vi "Server.vi"() -> ()   [LabVIEW 2020]
panel:
  in  "Door Stop":bool
  out "Open Door":bool
  out "Fire Alarm":bool
  out "AC4":bool
  out "AC3":bool
  out "AC2":bool
  out "AC1":bool
  out "KCW1":dbl(slide) scale=0.0..100.0
  out "KCW2":dbl(slide) scale=0.0..100.0
  out "B3W2":dbl(slide) scale=0.0..100.0
  out "B3W1":dbl(slide) scale=0.0..100.0
  out "B2W2":dbl(slide) scale=0.0..100.0
  out "B2W1":dbl(slide) scale=0.0..100.0
  out "LAW":dbl(slide) scale=0.0..100.0
  out "MBW":dbl(slide) scale=0.0..100.0
  out "MBC":bool
  out "B1C":bool
  out "MDC":bool
  out "B2C":bool
  out "B3C":bool
  out "TBC":bool
  out "SLC":bool
  out "B3O":bool
  out "B1O":bool
  out "LA":bool
  out "MBO":bool
  out "B2O":bool
  out "MDO":bool
  out "SLO":bool
  out "TBO":bool
  out "B3L2":bool
  out "B3L1":bool
  out "LL":bool
  out "B2WICL":bool
  out "B2L2":bool
  out "B2L1":bool
  out "MBL2":bool
  out "MBL1":bool
  out "GL2":bool
  out "GL1":bool
  out "MBWICL":bool
  out "MBL":bool
  out "KL2":bool
  out "KL1":bool
  out "TBL":bool
  out "SLL1":bool
  out "SLL2":bool
  out "DAL2":bool
  out "DAL1":bool
  out "LAL2":bool
  out "LAL1":bool
  out "PL":bool
  out "Brightness\nMaster Bath \nLight":u8
  out "Brightness\nKitchen \nLight 1":u8
  out "Brightness\nKitchen \nLight 2":u8
  out "Brightness\nService Laundry \nLight 1":u8
  out "Brightness\nService Laundry \nLight 2":u8
  out "Brightness\nT&B Light":u8
  out "Brightness\nMaster Bedroom \nLight 2":u8
  out "Brightness\nMaster Bedroom \nW.I.C. Light":u8
  out "Brightness\nLiving Area Light 1":u8
  out "Brightness\nLiving Area Light 2":u8
  out "Brightness\n Porch Light":u8
  out "Brightness\nBedroom 2 \nLight 2":u8
  out "Brightness\nBedroom 2 \nLight 1":u8
  out "Brightness\nLanai Light":u8
  out "Brightness\nDining Area Light 2":u8
  out "Brightness\nDining Area Light 1":u8
  out "Brightness\nGarage Light 2":u8
  out "Brightness\nGarage Light 1":u8
  out "Brightness\nBedroom 3 \nLight 2":u8
  out "Brightness\nBedroom 3 \nLight 1":u8
  out "Brightness\nBedroom 2 \nW.I.C. Light":u8
  out "Temperature":u8
  out "Brightness\nMaster Bedroom \nLight 1":u8
  in  "Alarm Stop":bool
  in  "Holiday Stop":bool
  in  "TV Living Area":refnum<k7>(container)
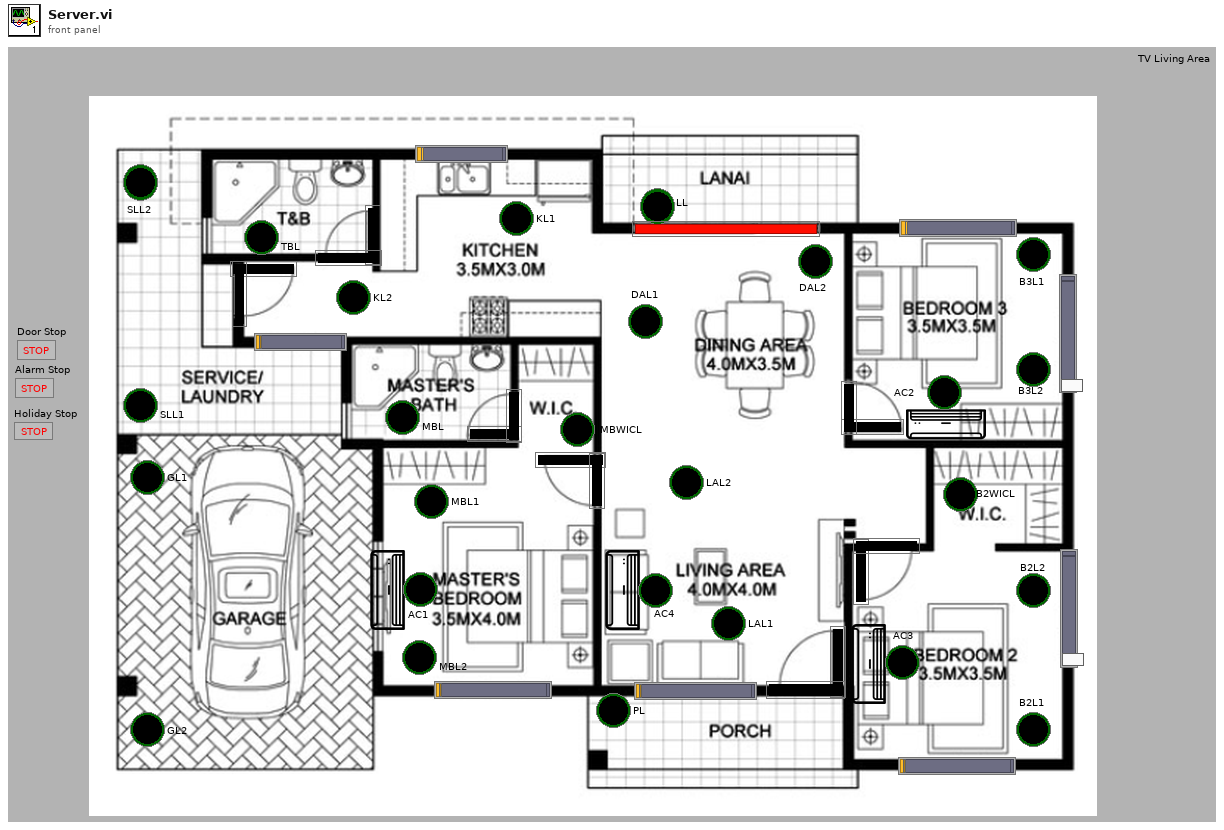
[diagram p1: front panel]
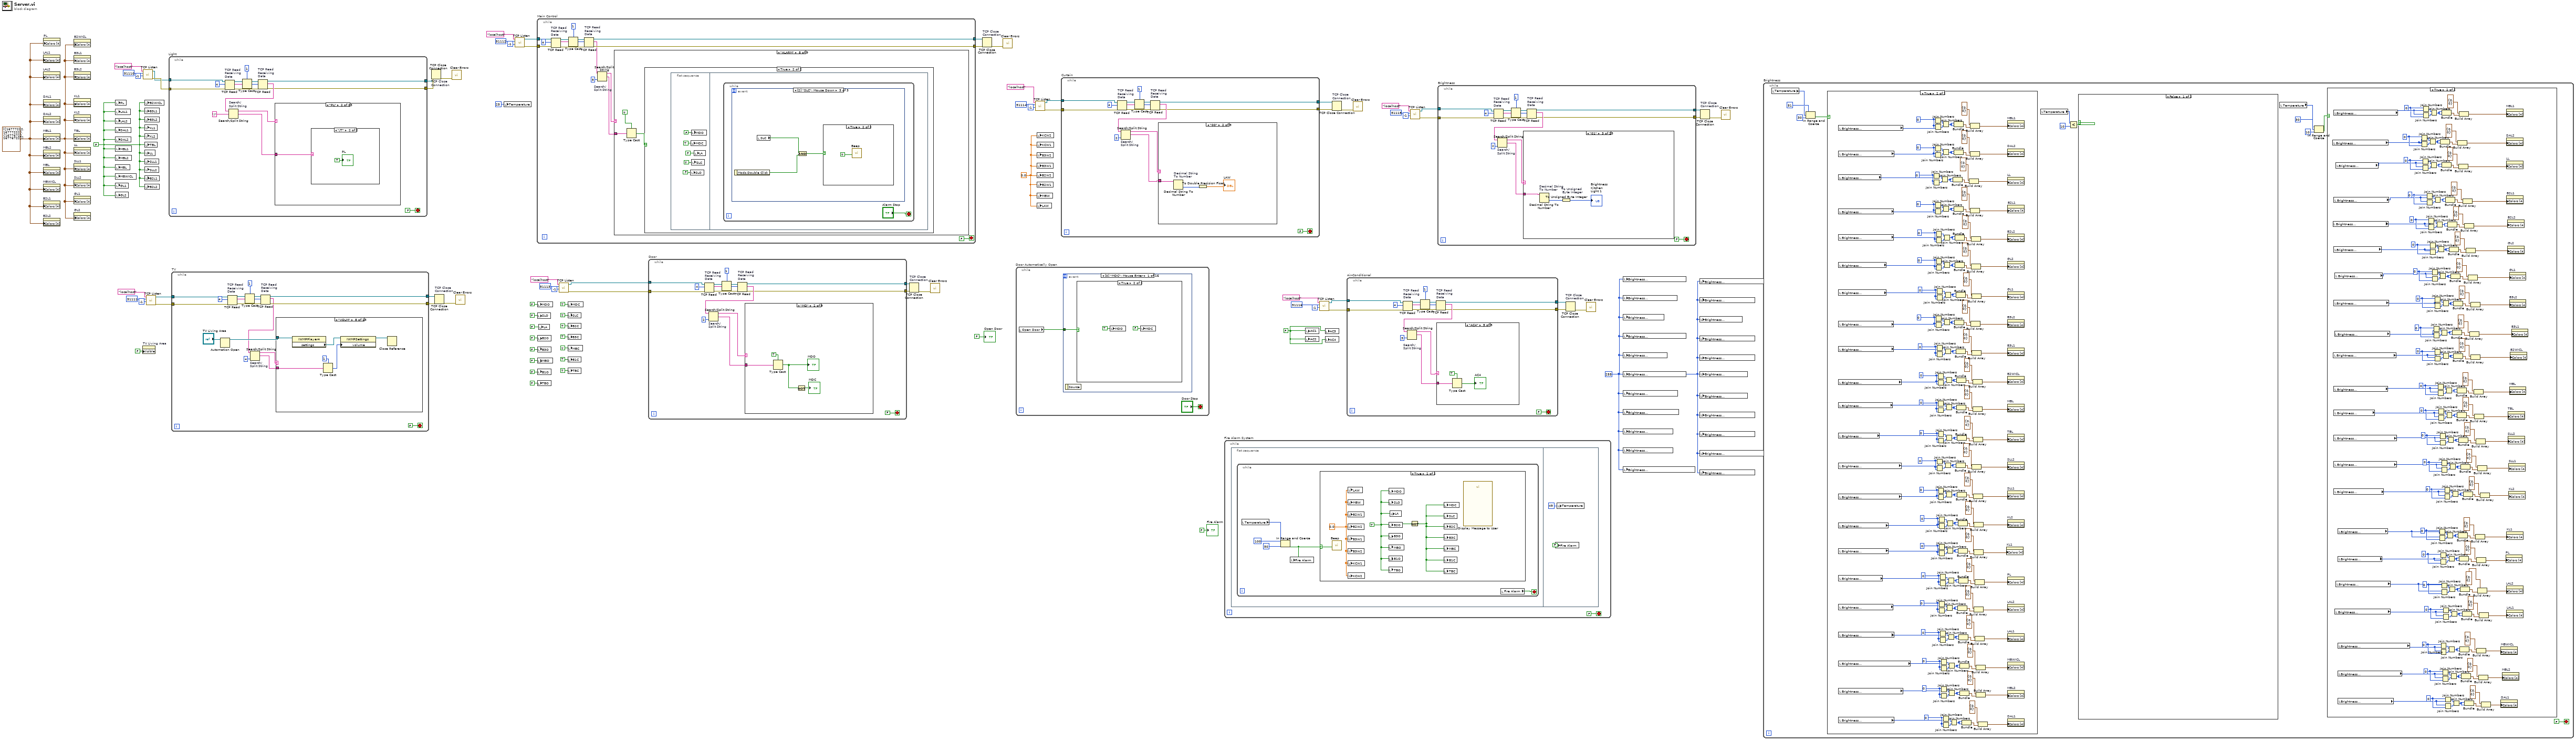
[diagram p0: block diagram]
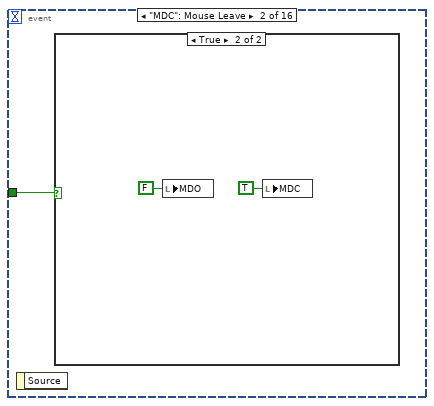
[diagram p3: hidden frame]
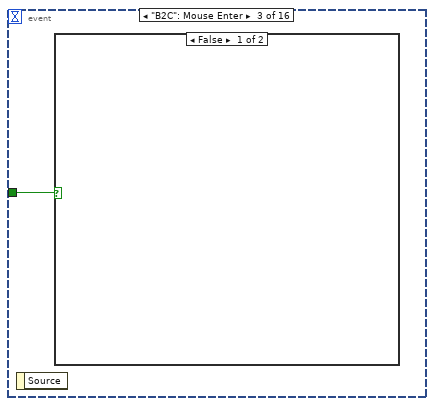
[diagram p5: hidden frame]
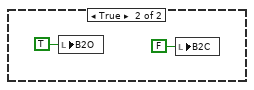
[diagram p6: hidden frame]
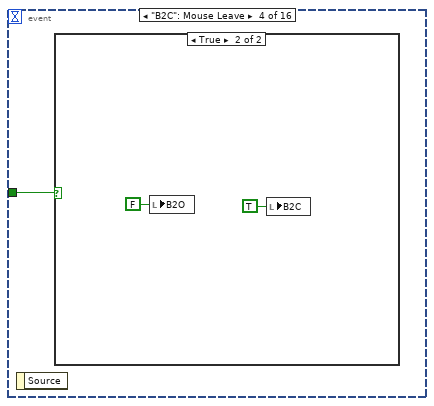
[diagram p7: hidden frame]
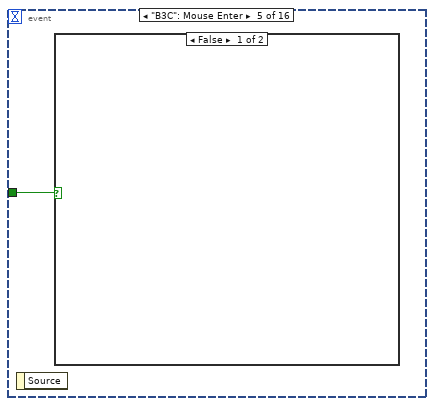
[diagram p9: hidden frame]
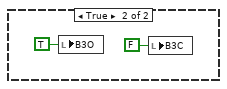
[diagram p10: hidden frame]
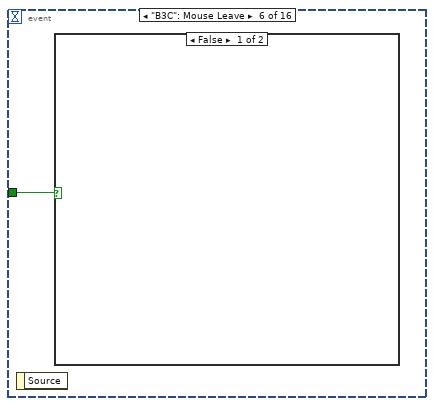
[diagram p11: hidden frame]
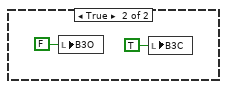
[diagram p12: hidden frame]
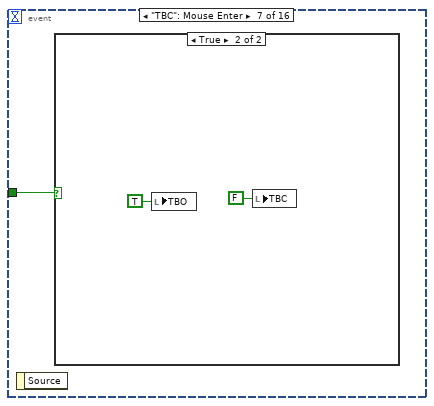
[diagram p13: hidden frame]
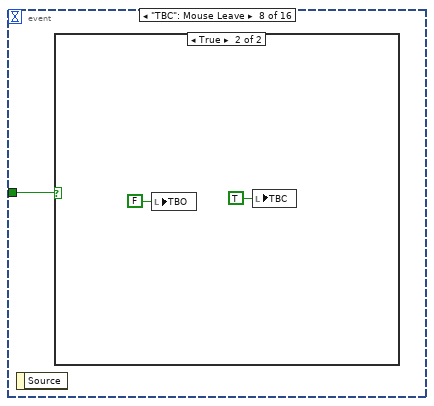
[diagram p15: hidden frame]
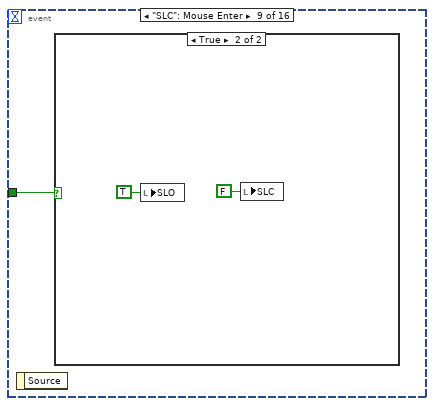
[diagram p17: hidden frame]
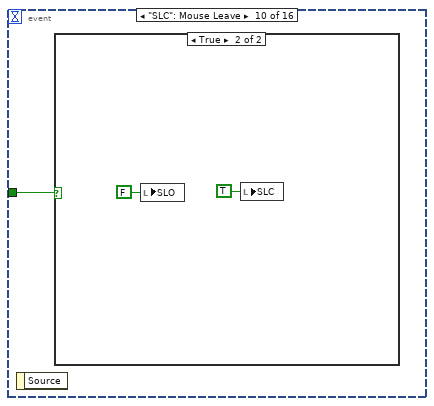
[diagram p19: hidden frame]
diagram:
  w3 = 0.0 ("B2W2")
  w4 = FALSE ("AC1")
  w13 = u8 255 ("Brightness\nService Laundry \nLight 1")
  w14 = cluster{u32, u32}[] [{16777222, 16777222}, {16776722, 16776722}] ("Colors [4]")
  w24 = FALSE
  n1 = property on="LAL1" class="Bool (strict)"("Colors [4]"=w14) -> ()  [unwired: 2 in, 2 out]
  n2 = property on="LAL2" class="Bool (strict)"("Colors [4]"=w14) -> ()  [unwired: 2 in, 2 out]
  n3 = property on="DAL1" class="Bool (strict)"("Colors [4]"=w14) -> ()  [unwired: 2 in, 2 out]
  n4 = property on="DAL2" class="Bool (strict)"("Colors [4]"=w14) -> ()  [unwired: 2 in, 2 out]
  n5 = property on="MBL1" class="Bool (strict)"("Colors [4]"=w14) -> ()  [unwired: 2 in, 2 out]
  n6 = property on="MBL2" class="Bool (strict)"("Colors [4]"=w14) -> ()  [unwired: 2 in, 2 out]
  n7 = property on="MBL" class="Bool (strict)"("Colors [4]"=w14) -> ()  [unwired: 2 in, 2 out]
  n8 = property on="MBWICL" class="Bool (strict)"("Colors [4]"=w14) -> ()  [unwired: 2 in, 2 out]
  n9 = property on="B2L1" class="Bool (strict)"("Colors [4]"=w14) -> ()  [unwired: 2 in, 2 out]
  n10 = property on="B2L2" class="Bool (strict)"("Colors [4]"=w14) -> ()  [unwired: 2 in, 2 out]
  n11 = property on="PL" class="Bool (strict)"("Colors [4]"=w14) -> ()  [unwired: 2 in, 2 out]
  n12 = property on="B2WICL" class="Bool (strict)"("Colors [4]"=w14) -> ()  [unwired: 2 in, 2 out]
  n13 = property on="B3L1" class="Bool (strict)"("Colors [4]"=w14) -> ()  [unwired: 2 in, 2 out]
  n14 = property on="B3L2" class="Bool (strict)"("Colors [4]"=w14) -> ()  [unwired: 2 in, 2 out]
  n15 = property on="KL1" class="Bool (strict)"("Colors [4]"=w14) -> ()  [unwired: 2 in, 2 out]
  n16 = property on="KL2" class="Bool (strict)"("Colors [4]"=w14) -> ()  [unwired: 2 in, 2 out]
  n17 = property on="TBL" class="Bool (strict)"("Colors [4]"=w14) -> ()  [unwired: 2 in, 2 out]
  n18 = property on="LL" class="Bool (strict)"("Colors [4]"=w14) -> ()  [unwired: 2 in, 2 out]
  n19 = property on="SLL1" class="Bool (strict)"("Colors [4]"=w14) -> ()  [unwired: 2 in, 2 out]
  n20 = property on="SLL2" class="Bool (strict)"("Colors [4]"=w14) -> ()  [unwired: 2 in, 2 out]
  n21 = property on="GL1" class="Bool (strict)"("Colors [4]"=w14) -> ()  [unwired: 2 in, 2 out]
  n22 = property on="GL2" class="Bool (strict)"("Colors [4]"=w14) -> ()  [unwired: 2 in, 2 out]
  n23 = local write "PL"(w24) -> ()
  n24 = local write "LAL1"(w24) -> ()
  n25 = local write "LAL2"(w24) -> ()
  n26 = local write "DAL1"(w24) -> ()
  n27 = local write "DAL2"(w24) -> ()
  n28 = local write "MBL1"(w24) -> ()
  n29 = local write "MBL2"(w24) -> ()
  n30 = local write "MBL"(w24) -> ()
  n31 = local write "MBWICL"(w24) -> ()
  n32 = local write "GL1"(w24) -> ()
  n33 = local write "GL2"(w24) -> ()
  n34 = property on="TV Living Area" class="AXCont"("Visible"=FALSE) -> ()  [unwired: 2 in, 2 out]
  n35 = call <vilib>:"TCP Listen.vi"("timeout ms (wait forever: -1)"=-1 ("timeout ms (60000)"), "port"=u16 51110 ("remote port or service name"), "service name"="localhost") -> ("error out"=w77:errorcluster, "connection ID"=w76:refnum<k5>)  [unwired: 4 in, 3 out]
  n36 = local write "B2WICL"(w24) -> ()
  n37 = local write "B3L1"(w24) -> ()
  n38 = local write "B3L2"(w24) -> ()
  n39 = local write "KL1"(w24) -> ()
  n40 = local write "KL2"(w24) -> ()
  n41 = local write "TBL"(w24) -> ()
  n42 = local write "LL"(w24) -> ()
  n43 = local write "SLL1"(w24) -> ()
  n44 = local write "SLL2"(w24) -> ()
  n45 = local write "B2L1"(w24) -> ()
  n46 = local write "B2L2"(w24) -> ()
  n47 = call <vilib>:"TCP Listen.vi"("timeout ms (wait forever: -1)"=-1 ("timeout ms (60000)"), "port"=u16 51111 ("remote port or service name"), "service name"="localhost") -> ("error out"=w68:errorcluster, "connection ID"=w69:refnum<k5>)  [unwired: 4 in, 3 out]
  n48 = while "Light" {
    tunnel: w77 -> [w84]
    tunnel: w76 -> [w83]
    tunnel: [w82] -> w74
    tunnel: [w81] -> w73
    stop <- FALSE stop-if-true
    n49 = TCP Read "TCP Read\nReceiving\nData"(connection ID=w83, bytes to read=4, error in (no error)=w84) -> (connection ID out=w90:refnum<k5>, data out=w93:string, error out=w89:errorcluster)  [unwired: 2 in]
    n50 = Type Cast(type=1 ("bytes to read"), x=w93) -> (*(type *) &x=w91:i32)
    n51 = TCP Read "TCP Read\nReceiving\nData"(connection ID=w90, bytes to read=w91, error in (no error)=w89) -> (connection ID out=w81:refnum<k5>, data out=w87:string, error out=w82:errorcluster)  [unwired: 2 in]
    n52 = Search/Split String "Search/\nSplit String"(string=w87, search string/char (-)="/" ("regular expression")) -> (substring before match=w86:string, match + rest of string=w85:string)  [unwired: 1 in, 1 out]
    n53 = case shown="\"PL\"" w86 {
      tunnel: w85 -> [_ w96 w99 w102 w105 w108 w111 w114 w117 w120 w123 w126 w129 w132 w135 w138 w141 w144 w147 w150 w153 w156 w159]
      frame "False", Default {
      }
      frame "PL" {
        n54 = case shown="\"/T\"" w96 {
          frame "F", Default {
            n55 = local write "PL"(FALSE ("PL")) -> ()
          }
          frame "/T" {
            "PL" <- TRUE ("PL")
          }
        }
      }
      frame "LAL1" {
        n56 = case shown="\"F\", Default" w99 {
          frame "F", Default {
            n57 = local write "LAL1"(FALSE ("LAL1")) -> ()
          }
          frame "/T" {
            "LAL1" <- TRUE ("LAL1")
          }
        }
      }
      frame "LAL2" {
        n58 = case shown="\"/T\"" w102 {
          frame "F", Default {
            n59 = local write "LAL2"(FALSE ("LAL2")) -> ()
          }
          frame "/T" {
            "LAL2" <- TRUE ("LAL2")
          }
        }
      }
      frame "DAL1" {
        n60 = case shown="\"/T\"" w105 {
          frame "F", Default {
            n61 = local write "DAL1"(FALSE ("DAL1")) -> ()
          }
          frame "/T" {
            "DAL1" <- TRUE ("DAL1")
          }
        }
      }
      frame "DAL2" {
        n62 = case shown="\"/T\"" w108 {
          frame "F", Default {
            n63 = local write "DAL2"(FALSE ("DAL2")) -> ()
          }
          frame "/T" {
            "DAL2" <- TRUE ("DAL2")
          }
        }
      }
      frame "MBL1" {
        n64 = case shown="\"/T\"" w111 {
          frame "F", Default {
            n65 = local write "MBL1"(FALSE ("MBL1")) -> ()
          }
          frame "/T" {
            "MBL1" <- TRUE ("MBL1")
          }
        }
      }
      frame "MBL2" {
        n66 = case shown="\"/T\"" w114 {
          frame "F", Default {
            n67 = local write "MBL2"(FALSE ("MBL2")) -> ()
          }
          frame "/T" {
            "MBL2" <- TRUE ("MBL2")
          }
        }
      }
      frame "MBL" {
        n68 = case shown="\"/T\"" w117 {
          frame "F", Default {
            n69 = local write "MBL"(FALSE ("MBL")) -> ()
          }
          frame "/T" {
            "MBL" <- TRUE ("MBL")
          }
        }
      }
      frame "MBWICL" {
        n70 = case shown="\"/T\"" w120 {
          frame "F", Default {
            n71 = local write "MBWICL"(FALSE ("MBWICL")) -> ()
          }
          frame "/T" {
            "MBWICL" <- TRUE ("MBWICL")
          }
        }
      }
      frame "B2L1" {
        n72 = case shown="\"/T\"" w123 {
          frame "F", Default {
            n73 = local write "B2L1"(FALSE ("B2L1")) -> ()
          }
          frame "/T" {
            "B2L1" <- TRUE ("B2L1")
          }
        }
      }
      frame "B2L2" {
        n74 = case shown="\"/T\"" w126 {
          frame "F", Default {
            n75 = local write "B2L2"(FALSE ("B2L2")) -> ()
          }
          frame "/T" {
            "B2L2" <- TRUE ("B2L2")
          }
        }
      }
      frame "B2WICL" {
        n76 = case shown="\"/T\"" w129 {
          frame "F", Default {
            n77 = local write "B2WICL"(FALSE ("B2WICL")) -> ()
          }
          frame "/T" {
            "B2WICL" <- TRUE ("B2WICL")
          }
        }
      }
      frame "B3L1" {
        n78 = case shown="\"/T\"" w132 {
          frame "F", Default {
            n79 = local write "B3L1"(FALSE ("B3L1")) -> ()
          }
          frame "/T" {
            "B3L1" <- TRUE ("B3L1")
          }
        }
      }
      frame "B3L2" {
        n80 = case shown="\"/T\"" w135 {
          frame "F", Default {
            n81 = local write "B3L2"(FALSE ("B3L2")) -> ()
          }
          frame "/T" {
            "B3L2" <- TRUE ("B3L2")
          }
        }
      }
      frame "KL1" {
        n82 = case shown="\"/T\"" w138 {
          frame "F", Default {
            n83 = local write "KL1"(FALSE ("KL1")) -> ()
          }
          frame "/T" {
            "KL1" <- TRUE ("KL1")
          }
        }
      }
      frame "KL2" {
        n84 = case shown="\"/T\"" w141 {
          frame "F", Default {
            n85 = local write "KL2"(FALSE ("KL2")) -> ()
          }
          frame "/T" {
            "KL2" <- TRUE ("KL2")
          }
        }
      }
      frame "TBL" {
        n86 = case shown="\"F\", Default" w144 {
          frame "F", Default {
            n87 = local write "TBL"(FALSE ("TBL")) -> ()
          }
          frame "/T" {
            "TBL" <- TRUE ("TBL")
          }
        }
      }
      frame "LL" {
        n88 = case shown="\"/T\"" w147 {
          frame "F", Default {
            n89 = local write "LL"(FALSE ("LL")) -> ()
          }
          frame "/T" {
            "LL" <- TRUE ("LL")
          }
        }
      }
      frame "SLL1" {
        n90 = case shown="\"/T\"" w150 {
          frame "F", Default {
            n91 = local write "SLL1"(FALSE ("SLL1")) -> ()
          }
          frame "/T" {
            "SLL1" <- TRUE ("SLL1")
          }
        }
      }
      frame "SLL2" {
        n92 = case shown="\"/T\"" w153 {
          frame "F", Default {
            n93 = local write "SLL2"(FALSE ("SLL2")) -> ()
          }
          frame "/T" {
            "SLL2" <- TRUE ("SLL2")
          }
        }
      }
      frame "GL1" {
        n94 = case shown="\"/T\"" w156 {
          frame "F", Default {
            n95 = local write "GL1"(FALSE ("GL1")) -> ()
          }
          frame "/T" {
            "GL1" <- TRUE ("GL1")
          }
        }
      }
      frame "GL2" {
        n96 = case shown="\"/T\"" w159 {
          frame "F", Default {
            n97 = local write "GL2"(FALSE ("GL2")) -> ()
          }
          frame "/T" {
            "GL2" <- TRUE ("GL2")
          }
        }
      }
    }
  }
  n98 = while "TV" {
    tunnel: w68 -> [w171]
    tunnel: w69 -> [w170]
    tunnel: [w169] -> w71
    tunnel: [w168] -> w72
    stop <- FALSE stop-if-true
    n99 = Automation Open(Automation Refnum="TV Living Area") -> (Automation Refnum=w167:refnum<k7>)  [unwired: 3 in, 1 out]
    n100 = TCP Read "TCP Read\nReceiving\nData"(connection ID=w170, bytes to read=4, error in (no error)=w171) -> (connection ID out=w173:refnum<k5>, data out=w176:string, error out=w172:errorcluster)  [unwired: 2 in]
    n101 = Type Cast(type=1 ("bytes to read"), x=w176) -> (*(type *) &x=w174:i32)
    n102 = TCP Read "TCP Read\nReceiving\nData"(connection ID=w173, bytes to read=w174, error in (no error)=w172) -> (connection ID out=w168:refnum<k5>, data out=w164:string, error out=w169:errorcluster)  [unwired: 2 in]
    n103 = Search/Split String "Search/\nSplit String"(string=w164, offset (0)=4) -> (substring before match=w165:string, match + rest of string=w162:string)  [unwired: 1 in, 1 out]
    n104 = case shown="\"VOLM\"" w165 {
      tunnel: w167 -> [_ w179 w184 w186 w188 w191 w199 w205 w206 w211 w214 w217 w220]
      tunnel: w162 -> [_ _ _ _ _ _ w194 w202 _ _ _ _ _]
      frame "False", Default {
      }
      frame "ONOF" {
        n105 = property on="TV Living Area" class="AXCont"() -> ("Visible"=w180:bool)  [unwired: 2 in, 2 out]
        n106 = Not(x=w180) -> (.not. x?=w181:bool)
        n107 = Close Reference(reference=w179) -> ()  [unwired: 1 in, 1 out]
        n108 = property on="TV Living Area" class="AXCont"("Visible"=w181) -> ()  [unwired: 2 in, 2 out]
      }
      frame "PLAY" {
        n109 = property class="IWMPPlayer4"(reference=w184) -> ("controls"=w183:refnum<k7>)  [unwired: 1 in, 2 out]
        n110 = invoke class="IWMPControls" method="play"(reference=w183) -> (reference out=w182:refnum<k7>)  [unwired: 2 in, 2 out]
        n111 = Close Reference(reference=w182) -> ()  [unwired: 1 in, 1 out]
      }
      frame "PAUS" {
        n112 = property class="IWMPPlayer4"(reference=w186) -> ("controls"=w185:refnum<k7>)  [unwired: 1 in, 2 out]
        n113 = invoke class="IWMPControls" method="pause"(reference=w185) -> (reference out=w187:refnum<k7>)  [unwired: 2 in, 2 out]
        n114 = Close Reference(reference=w187) -> ()  [unwired: 1 in, 1 out]
      }
      frame "FFWD" {
        n115 = property class="IWMPPlayer4"(reference=w188) -> ("controls"=w190:refnum<k7>)  [unwired: 1 in, 2 out]
        n116 = invoke class="IWMPControls" method="fastForward"(reference=w190) -> (reference out=w189:refnum<k7>)  [unwired: 2 in, 2 out]
        n117 = Close Reference(reference=w189) -> ()  [unwired: 1 in, 1 out]
      }
      frame "FRWD" {
        n118 = property class="IWMPPlayer4"(reference=w191) -> ("controls"=w193:refnum<k7>)  [unwired: 1 in, 2 out]
        n119 = invoke class="IWMPControls" method="fastReverse"(reference=w193) -> (reference out=w192:refnum<k7>)  [unwired: 2 in, 2 out]
        n120 = Close Reference(reference=w192) -> ()  [unwired: 1 in, 1 out]
      }
      frame "MUTE" {
        n121 = property class="IWMPPlayer4"(reference=w199) -> ("settings"=w198:refnum<k7>)  [unwired: 1 in, 2 out]
        n122 = Type Cast(type=TRUE, x=w194) -> (*(type *) &x=w195:bool)
        n123 = property class="IWMPSettings"(reference=w198, "mute"=w195) -> (reference out=w197:refnum<k7>)  [unwired: 1 in, 1 out]
        n124 = Close Reference(reference=w197) -> ()  [unwired: 1 in, 1 out]
      }
      frame "VOLM" {
        n125 = property class="IWMPPlayer4"(reference=w205) -> ("settings"=w204:refnum<k7>)  [unwired: 1 in, 2 out]
        n126 = Type Cast(type=1 ("bytes to read"), x=w202) -> (*(type *) &x=w200:i32)
        n127 = property class="IWMPSettings"(reference=w204, "volume"=w200) -> (reference out=w203:refnum<k7>)  [unwired: 1 in, 1 out]
        n128 = Close Reference(reference=w203) -> ()  [unwired: 1 in, 1 out]
      }
      frame "STOP" {
        n129 = property class="IWMPPlayer4"(reference=w206) -> ("controls"=w208:refnum<k7>)  [unwired: 1 in, 2 out]
        n130 = invoke class="IWMPControls" method="stop"(reference=w208) -> (reference out=w207:refnum<k7>)  [unwired: 2 in, 2 out]
        n131 = Close Reference(reference=w207) -> ()  [unwired: 1 in, 1 out]
      }
      frame "C1" {
        n132 = property class="IWMPPlayer4"(reference=w211, "URL"="C:\\Users\\MSI\\Downloads\\1.mp4") -> (reference out=w210:refnum<k7>)  [unwired: 1 in, 1 out]
        n133 = Close Reference(reference=w210) -> ()  [unwired: 1 in, 1 out]
      }
      frame "C2" {
        n134 = property class="IWMPPlayer4"(reference=w214, "URL"="C:\\Users\\MSI\\Downloads\\2.mp4") -> (reference out=w213:refnum<k7>)  [unwired: 1 in, 1 out]
        n135 = Close Reference(reference=w213) -> ()  [unwired: 1 in, 1 out]
      }
      frame "C3" {
        n136 = property class="IWMPPlayer4"(reference=w217, "URL"="C:\\Users\\MSI\\Downloads\\3.mp4") -> (reference out=w216:refnum<k7>)  [unwired: 1 in, 1 out]
        n137 = Close Reference(reference=w216) -> ()  [unwired: 1 in, 1 out]
      }
      frame "C4" {
        n138 = property class="IWMPPlayer4"(reference=w220, "URL"="C:\\Users\\MSI\\Downloads\\4.mp4") -> (reference out=w219:refnum<k7>)  [unwired: 1 in, 1 out]
        n139 = Close Reference(reference=w219) -> ()  [unwired: 1 in, 1 out]
      }
    }
  }
  n140 = TCP Close Connection "TCP Close \nConnection"(connection ID=w73, error in (no error)=w74) -> (error out=w75:errorcluster)  [unwired: 1 in, 1 out]
  n141 = TCP Close Connection "TCP Close \nConnection"(connection ID=w72, error in (no error)=w71) -> (error out=w70:errorcluster)  [unwired: 1 in, 1 out]
  n142 = call <vilib>:"Clear Errors.vi"("error in (no error)"=w75) -> ()  [unwired: 5 in, 2 out]
  n143 = call <vilib>:"Clear Errors.vi"("error in (no error)"=w70) -> ()  [unwired: 5 in, 2 out]
  n144 = local write "Temperature"(u8 25 ("Temperature")) -> ()
  n145 = call <vilib>:"TCP Listen.vi"("timeout ms (wait forever: -1)"=-1 ("timeout ms (60000)"), "port"=u16 51112 ("remote port or service name"), "service name"="localhost") -> ("error out"=w57:errorcluster, "connection ID"=w59:refnum<k5>)  [unwired: 4 in, 3 out]
  n146 = while "Main Control" {
    tunnel: w59 -> [w229]
    tunnel: [w228] -> w58
    tunnel: w57 -> [w227]
    tunnel: [w226] -> w56
    stop <- FALSE stop-if-true
    n147 = TCP Read "TCP Read\nReceiving\nData"(connection ID=w229, bytes to read=4, error in (no error)=w227) -> (connection ID out=w233:refnum<k5>, data out=w235:string, error out=w232:errorcluster)  [unwired: 2 in]
    n148 = Type Cast(type=1 ("bytes to read"), x=w235) -> (*(type *) &x=w234:i32)
    n149 = TCP Read "TCP Read\nReceiving\nData"(connection ID=w233, bytes to read=w234, error in (no error)=w232) -> (connection ID out=w228:refnum<k5>, data out=w225:string, error out=w226:errorcluster)  [unwired: 2 in]
    n150 = Search/Split String "Search/\nSplit String"(string=w225, offset (0)=5) -> (substring before match=w222:string, match + rest of string=w221:string)  [unwired: 1 in, 1 out]
    n151 = case shown="\"ALARM\"" w222 {
      tunnel: w221 -> [_ w240 w256 w270 w274 w277 w282 w534 w556]
      frame "False", Default {
      }
      frame "TEMPE" {
        n152 = Decimal String To Number "Decimal String \nTo Number"(string=w240) -> (number=w241:i32)  [unwired: 2 in, 1 out]
        n153 = To Unsigned Byte Integer "To Unsigned\n Byte Integer"(number=w241) -> (unsigned 8bit integer=w238:u8)
        "Temperature" <- w238
        n154 = Less?(x=w238, y=u8 10) -> (x < y?=w236:bool)
        n155 = In Range and Coerce "In Range \nand Coerce"(upper limit=30, x=w238, lower limit=10) -> (In Range?=w245:bool)  [unwired: 1 out]
        n156 = In Range and Coerce(upper limit=51, x=w238, lower limit=30 ("y")) -> (In Range?=w239:bool)  [unwired: 1 out]
        n157 = case shown="True" w236 {
          frame False {
          }
          frame True {
            w252 = FALSE ("AC1")
            n158 = local write "AC1"(w252) -> ()
            n159 = local write "AC2"(w252) -> ()
            n160 = local write "AC3"(w252) -> ()
            n161 = local write "AC4"(w252) -> ()
          }
        }
        n162 = Select(t=cluster{u32, u32}[] [{16777222, 16777222}, {16776722, 16776722}] ("Colors [4]"), s=w245, f=cluster{u32, u32}[] [{16777222, 16777222}, {6618880, 6618880}] ("Colors [4]")) -> (s? t:f=w246:cluster{u32, u32}[])
        n163 = Select(t=cluster{u32, u32}[] [{16777222, 16777222}, {16714752, 16714752}] ("Colors [4]"), s=w239, f=w246) -> (s? t:f=w250:cluster{u32, u32}[])
        n164 = case shown="True" w239 {
          frame False {
          }
          frame True {
            w253 = TRUE ("AC1")
            n165 = local write "AC1"(w253) -> ()
            n166 = local write "AC2"(w253) -> ()
            n167 = local write "AC3"(w253) -> ()
            n168 = local write "AC4"(w253) -> ()
          }
        }
        n169 = property on="PL" class="Bool (strict)"("Colors [4]"=w250) -> ()  [unwired: 2 in, 2 out]
        n170 = property on="LAL1" class="Bool (strict)"("Colors [4]"=w250) -> ()  [unwired: 2 in, 2 out]
        n171 = property on="LAL2" class="Bool (strict)"("Colors [4]"=w250) -> ()  [unwired: 2 in, 2 out]
        n172 = property on="DAL1" class="Bool (strict)"("Colors [4]"=w250) -> ()  [unwired: 2 in, 2 out]
        n173 = property on="DAL2" class="Bool (strict)"("Colors [4]"=w250) -> ()  [unwired: 2 in, 2 out]
        n174 = property on="MBL1" class="Bool (strict)"("Colors [4]"=w250) -> ()  [unwired: 2 in, 2 out]
        n175 = property on="MBL2" class="Bool (strict)"("Colors [4]"=w250) -> ()  [unwired: 2 in, 2 out]
        n176 = property on="MBL" class="Bool (strict)"("Colors [4]"=w250) -> ()  [unwired: 2 in, 2 out]
        n177 = property on="MBWICL" class="Bool (strict)"("Colors [4]"=w250) -> ()  [unwired: 2 in, 2 out]
        n178 = property on="B2L1" class="Bool (strict)"("Colors [4]"=w250) -> ()  [unwired: 2 in, 2 out]
        n179 = property on="B2L2" class="Bool (strict)"("Colors [4]"=w250) -> ()  [unwired: 2 in, 2 out]
        n180 = property on="B2WICL" class="Bool (strict)"("Colors [4]"=w250) -> ()  [unwired: 2 in, 2 out]
        n181 = property on="B3L1" class="Bool (strict)"("Colors [4]"=w250) -> ()  [unwired: 2 in, 2 out]
        n182 = property on="B3L2" class="Bool (strict)"("Colors [4]"=w250) -> ()  [unwired: 2 in, 2 out]
        n183 = property on="KL1" class="Bool (strict)"("Colors [4]"=w250) -> ()  [unwired: 2 in, 2 out]
        n184 = property on="KL2" class="Bool (strict)"("Colors [4]"=w250) -> ()  [unwired: 2 in, 2 out]
        n185 = property on="TBL" class="Bool (strict)"("Colors [4]"=w250) -> ()  [unwired: 2 in, 2 out]
        n186 = property on="LL" class="Bool (strict)"("Colors [4]"=w250) -> ()  [unwired: 2 in, 2 out]
        n187 = property on="SLL1" class="Bool (strict)"("Colors [4]"=w250) -> ()  [unwired: 2 in, 2 out]
        n188 = property on="SLL2" class="Bool (strict)"("Colors [4]"=w250) -> ()  [unwired: 2 in, 2 out]
        n189 = property on="GL1" class="Bool (strict)"("Colors [4]"=w250) -> ()  [unwired: 2 in, 2 out]
        n190 = property on="GL2" class="Bool (strict)"("Colors [4]"=w250) -> ()  [unwired: 2 in, 2 out]
      }
      frame "CLOCK" {
        n191 = Type Cast(type=TRUE, x=w256) -> (*(type *) &x=w254:bool)
        n192 = case shown="True" w254 {
          frame False {
            w257 = 100.0 ("B2W2")
            n193 = local read "TV Living Area"() -> (w262:refnum<k7>)
            n194 = Automation Open(Automation Refnum=w262) -> (Automation Refnum=w261:refnum<k7>)  [unwired: 3 in, 1 out]
            n195 = property class="IWMPPlayer4"(reference=w261) -> ("settings"=w260:refnum<k7>)  [unwired: 1 in, 2 out]
            n196 = local write "LAW"(w257) -> ()
            n197 = local write "MBW"(w257) -> ()
            n198 = local write "B2W1"(w257) -> ()
            n199 = local write "B2W2"(w257) -> ()
            n200 = local write "B3W1"(w257) -> ()
            n201 = local write "B3W2"(w257) -> ()
            n202 = local write "KCW1"(w257) -> ()
            n203 = local write "KCW2"(w257) -> ()
            n204 = property class="IWMPSettings"(reference=w260, "volume"=20) -> (reference out=w259:refnum<k7>)  [unwired: 1 in, 1 out]
            n205 = Close Reference(reference=w259) -> ()  [unwired: 1 in, 1 out]
          }
          frame True {
            w268 = 0.0 ("B2W2")
            n206 = local read "TV Living Area"() -> (w267:refnum<k7>)
            n207 = Automation Open(Automation Refnum=w267) -> (Automation Refnum=w266:refnum<k7>)  [unwired: 3 in, 1 out]
            n208 = property class="IWMPPlayer4"(reference=w266) -> ("settings"=w265:refnum<k7>)  [unwired: 1 in, 2 out]
            n209 = local write "LAW"(w268) -> ()
            n210 = local write "MBW"(w268) -> ()
            n211 = local write "B2W1"(w268) -> ()
            n212 = local write "B2W2"(w268) -> ()
            n213 = local write "B3W1"(w268) -> ()
            n214 = local write "B3W2"(w268) -> ()
            n215 = local write "KCW1"(w268) -> ()
            n216 = local write "KCW2"(w268) -> ()
            n217 = property class="IWMPSettings"(reference=w265, "volume"=50) -> (reference out=w264:refnum<k7>)  [unwired: 1 in, 1 out]
            n218 = Close Reference(reference=w264) -> ()  [unwired: 1 in, 1 out]
          }
        }
      }
      frame "MAINL" {
        n219 = Type Cast(type=TRUE, x=w270) -> (*(type *) &x=w269:bool)
        n220 = local write "PL"(w269) -> ()
        n221 = local write "LAL1"(w269) -> ()
        n222 = local write "LAL2"(w269) -> ()
        n223 = local write "DAL1"(w269) -> ()
        n224 = local write "DAL2"(w269) -> ()
        n225 = local write "MBL1"(w269) -> ()
        n226 = local write "MBL2"(w269) -> ()
        n227 = local write "MBL"(w269) -> ()
        n228 = local write "MBWICL"(w269) -> ()
        n229 = local write "B2WICL"(w269) -> ()
        n230 = local write "B3L1"(w269) -> ()
        n231 = local write "B3L2"(w269) -> ()
        n232 = local write "KL1"(w269) -> ()
        n233 = local write "KL2"(w269) -> ()
        n234 = local write "TBL"(w269) -> ()
        n235 = local write "LL"(w269) -> ()
        n236 = local write "SLL1"(w269) -> ()
        n237 = local write "SLL2"(w269) -> ()
        n238 = local write "B2L1"(w269) -> ()
        n239 = local write "B2L2"(w269) -> ()
        n240 = local write "GL1"(w269) -> ()
        n241 = local write "GL2"(w269) -> ()
      }
      frame "MAIND" {
        n242 = Type Cast(type=TRUE, x=w274) -> (*(type *) &x=w273:bool)
        n243 = local write "MDO"(w273) -> ()
        n244 = local write "SLO"(w273) -> ()
        n245 = local write "B2O"(w273) -> ()
        n246 = local write "B3O"(w273) -> ()
        n247 = local write "MBO"(w273) -> ()
        n248 = local write "B1O"(w273) -> ()
        n249 = local write "TBO"(w273) -> ()
        n250 = local write "LA"(w273) -> ()
        n251 = Not(x=w273) -> (.not. x?=w272:bool)
        n252 = local write "MDC"(w272) -> ()
        n253 = local write "SLC"(w272) -> ()
        n254 = local write "B2C"(w272) -> ()
        n255 = local write "B3C"(w272) -> ()
        n256 = local write "MBC"(w272) -> ()
        n257 = local write "B1C"(w272) -> ()
        n258 = local write "TBC"(w272) -> ()
      }
      frame "MAINW" {
        n259 = Type Cast(type=TRUE, x=w277) -> (*(type *) &x=w276:bool)
        n260 = case shown="True" w276 {
          frame False {
            w279 = 0.0 ("B2W2")
            n261 = local write "LAW"(w279) -> ()
            n262 = local write "MBW"(w279) -> ()
            n263 = local write "B2W1"(w279) -> ()
            n264 = local write "B2W2"(w279) -> ()
            n265 = local write "B3W1"(w279) -> ()
            n266 = local write "B3W2"(w279) -> ()
            n267 = local write "KCW1"(w279) -> ()
            n268 = local write "KCW2"(w279) -> ()
          }
          frame True {
            w280 = 100.0 ("B2W2")
            n269 = local write "LAW"(w280) -> ()
            n270 = local write "MBW"(w280) -> ()
            n271 = local write "B2W1"(w280) -> ()
            n272 = local write "B2W2"(w280) -> ()
            n273 = local write "B3W1"(w280) -> ()
            n274 = local write "B3W2"(w280) -> ()
            n275 = local write "KCW1"(w280) -> ()
            n276 = local write "KCW2"(w280) -> ()
          }
        }
      }
      frame "HLDMD" {
        n277 = Type Cast(type=FALSE, x=w282) -> (*(type *) &x=w281:bool)
        n278 = case shown="True" w281 {
          frame False {
            n279 = local write "PL"(FALSE ("PL")) -> ()
            n280 = local write "LAL1"(FALSE ("LAL1")) -> ()
            n281 = local write "LAL2"(FALSE ("LAL2")) -> ()
            n282 = local write "DAL1"(FALSE ("DAL1")) -> ()
            n283 = local write "DAL2"(FALSE ("DAL2")) -> ()
            n284 = local write "MBL1"(FALSE ("MBL1")) -> ()
            n285 = local write "MBL2"(FALSE ("MBL2")) -> ()
            n286 = local write "MBL"(FALSE ("MBL")) -> ()
            n287 = local write "MBWICL"(FALSE ("MBWICL")) -> ()
            n288 = local write "B2WICL"(FALSE ("B2WICL")) -> ()
            n289 = local write "B3L1"(FALSE ("B3L1")) -> ()
            n290 = local write "B3L2"(FALSE ("B3L2")) -> ()
            n291 = local write "KL1"(FALSE ("KL1")) -> ()
            n292 = local write "KL2"(FALSE ("KL2")) -> ()
            n293 = local write "TBL"(FALSE ("TBL")) -> ()
            n294 = local write "LL"(FALSE ("LL")) -> ()
            n295 = local write "SLL1"(FALSE ("SLL1")) -> ()
            n296 = local write "SLL2"(FALSE ("SLL2")) -> ()
            n297 = local write "B2L1"(FALSE ("B2L1")) -> ()
            n298 = local write "B2L2"(FALSE ("B2L2")) -> ()
            n299 = local write "GL1"(FALSE ("GL1")) -> ()
            n300 = local write "GL2"(FALSE ("GL2")) -> ()
          }
          frame True {
            n301 = while {
              stop <- "Holiday Stop" stop-if-true
              n302 = flat-sequence {
                frame #0 {
                  n303 = local write "PL"(FALSE ("PL")) -> ()
                  n304 = local write "LAL1"(FALSE ("LAL1")) -> ()
                  n305 = local write "LAL2"(FALSE ("LAL2")) -> ()
                  n306 = local write "DAL1"(FALSE ("DAL1")) -> ()
                  n307 = local write "DAL2"(FALSE ("DAL2")) -> ()
                  n308 = local write "MBL1"(FALSE ("MBL1")) -> ()
                  n309 = local write "MBL2"(FALSE ("MBL2")) -> ()
                  n310 = local write "MBL"(FALSE ("MBL")) -> ()
                  n311 = local write "MBWICL"(FALSE ("MBWICL")) -> ()
                  n312 = local write "B2WICL"(FALSE ("B2WICL")) -> ()
                  n313 = local write "B3L1"(FALSE ("B3L1")) -> ()
                  n314 = local write "B3L2"(FALSE ("B3L2")) -> ()
                  n315 = local write "KL1"(FALSE ("KL1")) -> ()
                  n316 = local write "KL2"(FALSE ("KL2")) -> ()
                  n317 = local write "TBL"(FALSE ("TBL")) -> ()
                  n318 = local write "LL"(FALSE ("LL")) -> ()
                  n319 = local write "SLL1"(FALSE ("SLL1")) -> ()
                  n320 = local write "SLL2"(FALSE ("SLL2")) -> ()
                  n321 = local write "B2L1"(FALSE ("B2L1")) -> ()
                  n322 = local write "B2L2"(FALSE ("B2L2")) -> ()
                  n323 = local write "GL1"(FALSE ("GL1")) -> ()
                  n324 = local write "GL2"(FALSE ("GL2")) -> ()
                }
                frame #1 {
                  n325 = Random Number (0-1) "Random \nNumber \n(0-1)"() -> (number: 0 to 1=w332:dbl)
                  n326 = Wait (ms)(milliseconds to wait=u32 1000) -> ()  [unwired: 1 out]
                  n327 = Multiply(x=10.0, y=w332) -> (x*y=w331:dbl)
                  n328 = Format Into String "Format Into String"(format string="%02d" ("initial string"), w331) -> (resulting string=w333:string)  [unwired: 2 in, 1 out]
                  n329 = case shown="\"10\"" w333 {
                    frame "00", Default {
                      n330 = local write "PL"(FALSE ("PL")) -> ()
                      n331 = local write "LAL1"(FALSE ("LAL1")) -> ()
                      n332 = local write "LAL2"(FALSE ("LAL2")) -> ()
                      n333 = local write "DAL1"(TRUE ("DAL1")) -> ()
                      n334 = local write "DAL2"(FALSE ("DAL2")) -> ()
                      n335 = local write "MBL1"(FALSE ("MBL1")) -> ()
                      n336 = local write "MBL2"(FALSE ("MBL2")) -> ()
                      n337 = local write "GL1"(FALSE ("GL1")) -> ()
                      n338 = local write "GL2"(FALSE ("GL2")) -> ()
                      n339 = local write "B3L1"(FALSE ("B3L1")) -> ()
                      n340 = local write "B3L2"(FALSE ("B3L2")) -> ()
                      n341 = local write "KL1"(TRUE ("KL1")) -> ()
                      n342 = local write "KL2"(FALSE ("KL2")) -> ()
                      n343 = local write "LL"(FALSE ("LL")) -> ()
                      n344 = local write "SLL1"(FALSE ("SLL1")) -> ()
                      n345 = local write "SLL2"(FALSE ("SLL2")) -> ()
                      n346 = local write "B2L1"(FALSE ("B2L1")) -> ()
                      n347 = local write "B2L2"(TRUE ("B2L2")) -> ()
                    }
                    frame "01" {
                      n348 = local write "PL"(FALSE ("PL")) -> ()
                      n349 = local write "LAL1"(FALSE ("LAL1")) -> ()
                      n350 = local write "LAL2"(FALSE ("LAL2")) -> ()
                      n351 = local write "DAL1"(FALSE ("DAL1")) -> ()
                      n352 = local write "DAL2"(TRUE ("DAL2")) -> ()
                      n353 = local write "MBL1"(FALSE ("MBL1")) -> ()
                      n354 = local write "MBL2"(TRUE ("MBL2")) -> ()
                      n355 = local write "GL1"(FALSE ("GL1")) -> ()
                      n356 = local write "GL2"(FALSE ("GL2")) -> ()
                      n357 = local write "B3L1"(TRUE ("B3L1")) -> ()
                      n358 = local write "B3L2"(FALSE ("B3L2")) -> ()
                      n359 = local write "KL1"(FALSE ("KL1")) -> ()
                      n360 = local write "KL2"(FALSE ("KL2")) -> ()
                      n361 = local write "LL"(FALSE ("LL")) -> ()
                      n362 = local write "SLL1"(FALSE ("SLL1")) -> ()
                      n363 = local write "SLL2"(FALSE ("SLL2")) -> ()
                      n364 = local write "B2L1"(FALSE ("B2L1")) -> ()
                      n365 = local write "B2L2"(FALSE ("B2L2")) -> ()
                    }
                    frame "02" {
                      n366 = local write "PL"(TRUE ("PL")) -> ()
                      n367 = local write "LAL1"(FALSE ("LAL1")) -> ()
                      n368 = local write "LAL2"(FALSE ("LAL2")) -> ()
                      n369 = local write "DAL1"(FALSE ("DAL1")) -> ()
                      n370 = local write "DAL2"(FALSE ("DAL2")) -> ()
                      n371 = local write "MBL1"(FALSE ("MBL1")) -> ()
                      n372 = local write "MBL2"(FALSE ("MBL2")) -> ()
                      n373 = local write "GL1"(TRUE ("GL1")) -> ()
                      n374 = local write "GL2"(FALSE ("GL2")) -> ()
                      n375 = local write "B3L1"(FALSE ("B3L1")) -> ()
                      n376 = local write "B3L2"(FALSE ("B3L2")) -> ()
                      n377 = local write "KL1"(TRUE ("KL1")) -> ()
                      n378 = local write "KL2"(FALSE ("KL2")) -> ()
                      n379 = local write "LL"(FALSE ("LL")) -> ()
                      n380 = local write "SLL1"(FALSE ("SLL1")) -> ()
                      n381 = local write "SLL2"(FALSE ("SLL2")) -> ()
                      n382 = local write "B2L1"(FALSE ("B2L1")) -> ()
                      n383 = local write "B2L2"(FALSE ("B2L2")) -> ()
                    }
                    frame "03" {
                      n384 = local write "PL"(FALSE ("PL")) -> ()
                      n385 = local write "LAL1"(TRUE ("LAL1")) -> ()
                      n386 = local write "LAL2"(FALSE ("LAL2")) -> ()
                      n387 = local write "DAL1"(FALSE ("DAL1")) -> ()
                      n388 = local write "DAL2"(TRUE ("DAL2")) -> ()
                      n389 = local write "MBL1"(FALSE ("MBL1")) -> ()
                      n390 = local write "MBL2"(FALSE ("MBL2")) -> ()
                      n391 = local write "GL1"(FALSE ("GL1")) -> ()
                      n392 = local write "GL2"(FALSE ("GL2")) -> ()
                      n393 = local write "B3L1"(TRUE ("B3L1")) -> ()
                      n394 = local write "B3L2"(FALSE ("B3L2")) -> ()
                      n395 = local write "KL1"(FALSE ("KL1")) -> ()
                      n396 = local write "KL2"(FALSE ("KL2")) -> ()
                      n397 = local write "LL"(FALSE ("LL")) -> ()
                      n398 = local write "SLL1"(FALSE ("SLL1")) -> ()
                      n399 = local write "SLL2"(FALSE ("SLL2")) -> ()
                      n400 = local write "B2L1"(FALSE ("B2L1")) -> ()
                      n401 = local write "B2L2"(FALSE ("B2L2")) -> ()
                    }
                    frame "04" {
                      n402 = local write "PL"(TRUE ("PL")) -> ()
                      n403 = local write "LAL1"(FALSE ("LAL1")) -> ()
                      n404 = local write "LAL2"(FALSE ("LAL2")) -> ()
                      n405 = local write "DAL1"(FALSE ("DAL1")) -> ()
                      n406 = local write "DAL2"(FALSE ("DAL2")) -> ()
                      n407 = local write "MBL1"(FALSE ("MBL1")) -> ()
                      n408 = local write "MBL2"(FALSE ("MBL2")) -> ()
                      n409 = local write "GL1"(FALSE ("GL1")) -> ()
                      n410 = local write "GL2"(TRUE ("GL2")) -> ()
                      n411 = local write "B3L1"(FALSE ("B3L1")) -> ()
                      n412 = local write "B3L2"(TRUE ("B3L2")) -> ()
                      n413 = local write "KL1"(FALSE ("KL1")) -> ()
                      n414 = local write "KL2"(FALSE ("KL2")) -> ()
                      n415 = local write "LL"(FALSE ("LL")) -> ()
                      n416 = local write "SLL1"(FALSE ("SLL1")) -> ()
                      n417 = local write "SLL2"(FALSE ("SLL2")) -> ()
                      n418 = local write "B2L1"(FALSE ("B2L1")) -> ()
                      n419 = local write "B2L2"(FALSE ("B2L2")) -> ()
                    }
                    frame "05" {
                      n420 = local write "PL"(FALSE ("PL")) -> ()
                      n421 = local write "LAL1"(FALSE ("LAL1")) -> ()
                      n422 = local write "LAL2"(FALSE ("LAL2")) -> ()
                      n423 = local write "DAL1"(FALSE ("DAL1")) -> ()
                      n424 = local write "DAL2"(FALSE ("DAL2")) -> ()
                      n425 = local write "MBL1"(FALSE ("MBL1")) -> ()
                      n426 = local write "MBL2"(TRUE ("MBL2")) -> ()
                      n427 = local write "GL1"(FALSE ("GL1")) -> ()
                      n428 = local write "GL2"(FALSE ("GL2")) -> ()
                      n429 = local write "B3L1"(FALSE ("B3L1")) -> ()
                      n430 = local write "B3L2"(FALSE ("B3L2")) -> ()
                      n431 = local write "KL1"(FALSE ("KL1")) -> ()
                      n432 = local write "KL2"(FALSE ("KL2")) -> ()
                      n433 = local write "LL"(TRUE ("LL")) -> ()
                      n434 = local write "SLL1"(TRUE ("SLL1")) -> ()
                      n435 = local write "SLL2"(FALSE ("SLL2")) -> ()
                      n436 = local write "B2L1"(FALSE ("B2L1")) -> ()
                      n437 = local write "B2L2"(FALSE ("B2L2")) -> ()
                    }
                    frame "06" {
                      n438 = local write "PL"(FALSE ("PL")) -> ()
                      n439 = local write "LAL1"(FALSE ("LAL1")) -> ()
                      n440 = local write "LAL2"(TRUE ("LAL2")) -> ()
                      n441 = local write "DAL1"(FALSE ("DAL1")) -> ()
                      n442 = local write "DAL2"(FALSE ("DAL2")) -> ()
                      n443 = local write "MBL1"(TRUE ("MBL1")) -> ()
                      n444 = local write "MBL2"(FALSE ("MBL2")) -> ()
                      n445 = local write "GL1"(FALSE ("GL1")) -> ()
                      n446 = local write "GL2"(FALSE ("GL2")) -> ()
                      n447 = local write "B3L1"(FALSE ("B3L1")) -> ()
                      n448 = local write "B3L2"(FALSE ("B3L2")) -> ()
                      n449 = local write "KL1"(FALSE ("KL1")) -> ()
                      n450 = local write "KL2"(FALSE ("KL2")) -> ()
                      n451 = local write "LL"(FALSE ("LL")) -> ()
                      n452 = local write "SLL1"(FALSE ("SLL1")) -> ()
                      n453 = local write "SLL2"(FALSE ("SLL2")) -> ()
                      n454 = local write "B2L1"(TRUE ("B2L1")) -> ()
                      n455 = local write "B2L2"(FALSE ("B2L2")) -> ()
                    }
                    frame "07" {
                      n456 = local write "PL"(FALSE ("PL")) -> ()
                      n457 = local write "LAL1"(TRUE ("LAL1")) -> ()
                      n458 = local write "LAL2"(FALSE ("LAL2")) -> ()
                      n459 = local write "DAL1"(FALSE ("DAL1")) -> ()
                      n460 = local write "DAL2"(TRUE ("DAL2")) -> ()
                      n461 = local write "MBL1"(FALSE ("MBL1")) -> ()
                      n462 = local write "MBL2"(FALSE ("MBL2")) -> ()
                      n463 = local write "GL1"(FALSE ("GL1")) -> ()
                      n464 = local write "GL2"(FALSE ("GL2")) -> ()
                      n465 = local write "B3L1"(TRUE ("B3L1")) -> ()
                      n466 = local write "B3L2"(FALSE ("B3L2")) -> ()
                      n467 = local write "KL1"(FALSE ("KL1")) -> ()
                      n468 = local write "KL2"(FALSE ("KL2")) -> ()
                      n469 = local write "LL"(FALSE ("LL")) -> ()
                      n470 = local write "SLL1"(FALSE ("SLL1")) -> ()
                      n471 = local write "SLL2"(FALSE ("SLL2")) -> ()
                      n472 = local write "B2L1"(FALSE ("B2L1")) -> ()
                      n473 = local write "B2L2"(FALSE ("B2L2")) -> ()
                    }
                    frame "08" {
                      n474 = local write "PL"(TRUE ("PL")) -> ()
                      n475 = local write "LAL1"(FALSE ("LAL1")) -> ()
                      n476 = local write "LAL2"(FALSE ("LAL2")) -> ()
                      n477 = local write "DAL1"(FALSE ("DAL1")) -> ()
                      n478 = local write "DAL2"(FALSE ("DAL2")) -> ()
                      n479 = local write "MBL1"(FALSE ("MBL1")) -> ()
                      n480 = local write "MBL2"(FALSE ("MBL2")) -> ()
                      n481 = local write "GL1"(FALSE ("GL1")) -> ()
                      n482 = local write "GL2"(TRUE ("GL2")) -> ()
                      n483 = local write "B3L1"(FALSE ("B3L1")) -> ()
                      n484 = local write "B3L2"(FALSE ("B3L2")) -> ()
                      n485 = local write "KL1"(FALSE ("KL1")) -> ()
                      n486 = local write "KL2"(FALSE ("KL2")) -> ()
                      n487 = local write "LL"(TRUE ("LL")) -> ()
                      n488 = local write "SLL1"(FALSE ("SLL1")) -> ()
                      n489 = local write "SLL2"(FALSE ("SLL2")) -> ()
                      n490 = local write "B2L1"(FALSE ("B2L1")) -> ()
                      n491 = local write "B2L2"(FALSE ("B2L2")) -> ()
                    }
                    frame "09" {
                      n492 = local write "PL"(FALSE ("PL")) -> ()
                      n493 = local write "LAL1"(FALSE ("LAL1")) -> ()
                      n494 = local write "LAL2"(FALSE ("LAL2")) -> ()
                      n495 = local write "DAL1"(FALSE ("DAL1")) -> ()
                      n496 = local write "DAL2"(FALSE ("DAL2")) -> ()
                      n497 = local write "MBL1"(TRUE ("MBL1")) -> ()
                      n498 = local write "MBL2"(FALSE ("MBL2")) -> ()
                      n499 = local write "GL1"(FALSE ("GL1")) -> ()
                      n500 = local write "GL2"(FALSE ("GL2")) -> ()
                      n501 = local write "B3L1"(FALSE ("B3L1")) -> ()
                      n502 = local write "B3L2"(FALSE ("B3L2")) -> ()
                      n503 = local write "KL1"(FALSE ("KL1")) -> ()
                      n504 = local write "KL2"(FALSE ("KL2")) -> ()
                      n505 = local write "LL"(FALSE ("LL")) -> ()
                      n506 = local write "SLL1"(TRUE ("SLL1")) -> ()
                      n507 = local write "SLL2"(FALSE ("SLL2")) -> ()
                      n508 = local write "B2L1"(TRUE ("B2L1")) -> ()
                      n509 = local write "B2L2"(FALSE ("B2L2")) -> ()
                    }
                    frame "10" {
                      n510 = local write "PL"(FALSE ("PL")) -> ()
                      n511 = local write "LAL1"(FALSE ("LAL1")) -> ()
                      n512 = local write "LAL2"(FALSE ("LAL2")) -> ()
                      n513 = local write "DAL1"(TRUE ("DAL1")) -> ()
                      n514 = local write "DAL2"(FALSE ("DAL2")) -> ()
                      n515 = local write "MBL1"(FALSE ("MBL1")) -> ()
                      n516 = local write "MBL2"(FALSE ("MBL2")) -> ()
                      n517 = local write "GL1"(FALSE ("GL1")) -> ()
                      n518 = local write "GL2"(FALSE ("GL2")) -> ()
                      n519 = local write "B3L1"(FALSE ("B3L1")) -> ()
                      n520 = local write "B3L2"(FALSE ("B3L2")) -> ()
                      n521 = local write "KL1"(FALSE ("KL1")) -> ()
                      n522 = local write "KL2"(TRUE ("KL2")) -> ()
                      n523 = local write "LL"(FALSE ("LL")) -> ()
                      n524 = local write "SLL1"(FALSE ("SLL1")) -> ()
                      n525 = local write "SLL2"(TRUE ("SLL2")) -> ()
                      n526 = local write "B2L1"(FALSE ("B2L1")) -> ()
                      n527 = local write "B2L2"(FALSE ("B2L2")) -> ()
                    }
                  }
                }
              }
            }
          }
        }
      }
      frame "ALARM" {
        n528 = Type Cast(type=TRUE, x=w534) -> (*(type *) &x=w533:bool)
        n529 = case shown="True" w533 {
          frame False {
          }
          frame True {
            n530 = flat-sequence {
              frame #0 {
                n531 = local write "SLO"(FALSE ("SLO")) -> ()
                n532 = local write "MDC"(TRUE ("MDC")) -> ()
                n533 = local write "MDO"(FALSE ("MDO")) -> ()
                n534 = local write "SLC"(TRUE ("SLC")) -> ()
                n535 = local write "LA"(FALSE ("LAO")) -> ()
              }
              frame #1 {
                n536 = while {
                  stop <- "Alarm Stop" stop-if-true
                  n537 = event shown="[2] \"SLC\": Mouse Down" {
                    selector: _ -> [_ _ _]
                    dyn-events: _ -> [_ _ _]
                    timeout: _ -> [_ _ _]
                    event "MDC": Mouse Down {
                      n538 = event-data() -> ("Mods.Double Click"=w543:bool)  [unwired: 1 in]
                      n539 = local read "MDC"() -> (w544:bool)
                      n540 = And(x=w544, y=w543) -> (x .and. y?=w542:bool)
                      n541 = case shown="True" w542 {
                        frame False {
                        }
                        frame True {
                          n542 = call <vilib>:"Beep.vi"("use system alert? (T)"=TRUE) -> ()  [unwired: 11 in]
                        }
                      }
                    }
                    event "LA": Mouse Down {
                      n543 = event-data() -> ("Mods.Double Click"=w549:bool)  [unwired: 1 in]
                      n544 = local read "LA"() -> (w547:bool)
                      n545 = Not(x=w547) -> (.not. x?=w546:bool)
                      n546 = And(x=w546, y=w549) -> (x .and. y?=w548:bool)
                      n547 = case shown="True" w548 {
                        frame False {
                        }
                        frame True {
                          n548 = call <vilib>:"Beep.vi"("use system alert? (T)"=TRUE) -> ()  [unwired: 11 in]
                        }
                      }
                    }
                    event "SLC": Mouse Down {
                      n549 = event-data() -> ("Mods.Double Click"=w553:bool)  [unwired: 1 in]
                      n550 = local read "SLC"() -> (w551:bool)
                      n551 = And(x=w551, y=w553) -> (x .and. y?=w552:bool)
                      n552 = case shown="True" w552 {
                        frame False {
                        }
                        frame True {
                          n553 = call <vilib>:"Beep.vi"("use system alert? (T)"=TRUE) -> ()  [unwired: 11 in]
                        }
                      }
                    }
                  }
                }
              }
            }
          }
        }
      }
      frame "DRAOP" {
        n554 = Type Cast(type=TRUE, x=w556) -> (*(type *) &x=w555:bool)
        n555 = local write "Open Door"(w555) -> ()
      }
    }
  }
  n556 = local write "MDO"(FALSE ("MDO")) -> ()
  n557 = local write "SLO"(FALSE ("SLO")) -> ()
  n558 = local write "B2O"(FALSE ("B2O")) -> ()
  n559 = local write "B3O"(FALSE ("B3O")) -> ()
  n560 = local write "MBO"(FALSE ("MBO")) -> ()
  n561 = local write "B1O"(FALSE ("B1O")) -> ()
  n562 = local write "TBO"(FALSE ("TBO")) -> ()
  n563 = local write "LA"(FALSE ("LAO")) -> ()
  n564 = call <vilib>:"TCP Listen.vi"("timeout ms (wait forever: -1)"=-1 ("timeout ms (60000)"), "port"=u16 51113 ("remote port or service name"), "service name"="localhost") -> ("error out"=w52:errorcluster, "connection ID"=w51:refnum<k5>)  [unwired: 4 in, 3 out]
  n565 = local write "MDC"(TRUE ("MDC")) -> ()
  n566 = local write "SLC"(TRUE ("SLC")) -> ()
  n567 = local write "B2C"(TRUE ("B2C")) -> ()
  n568 = local write "B3C"(TRUE ("B3C")) -> ()
  n569 = local write "MBC"(TRUE ("MBC")) -> ()
  n570 = local write "B1C"(TRUE ("B1C")) -> ()
  n571 = local write "TBC"(TRUE ("TBC")) -> ()
  n572 = while "Door" {
    tunnel: w52 -> [w564]
    tunnel: w51 -> [w563]
    tunnel: [w562] -> w49
    tunnel: [w561] -> w48
    stop <- FALSE stop-if-true
    n573 = TCP Read "TCP Read\nReceiving\nData"(connection ID=w563, bytes to read=4, error in (no error)=w564) -> (connection ID out=w567:refnum<k5>, data out=w570:string, error out=w566:errorcluster)  [unwired: 2 in]
    n574 = Type Cast(type=1 ("bytes to read"), x=w570) -> (*(type *) &x=w568:i32)
    n575 = TCP Read "TCP Read\nReceiving\nData"(connection ID=w567, bytes to read=w568, error in (no error)=w566) -> (connection ID out=w561:refnum<k5>, data out=w565:string, error out=w562:errorcluster)  [unwired: 2 in]
    n576 = Search/Split String "Search/\nSplit String"(string=w565, offset (0)=2) -> (substring before match=w559:string, match + rest of string=w558:string)  [unwired: 1 in, 1 out]
    n577 = case shown="\"MD\"" w559 {
      tunnel: w558 -> [_ w575 w579 w582 w586 w591 w594 w598 w602]
      frame "False", Default {
      }
      frame "MD" {
        n578 = Type Cast(type=TRUE ("MDC"), x=w575) -> (*(type *) &x=w573:bool)
        "MDO" <- w573
        n579 = Not(x=w573) -> (.not. x?=→"MDC":bool)
      }
      frame "SL" {
        n580 = Type Cast(type=TRUE ("MDC"), x=w579) -> (*(type *) &x=w578:bool)
        "SLO" <- w578
        n581 = Not(x=w578) -> (.not. x?=→"SLC":bool)
      }
      frame "LA" {
        n582 = Type Cast(type=TRUE ("MDC"), x=w582) -> (*(type *) &x=→"LA":bool)
      }
      frame "B2" {
        n583 = Type Cast(type=TRUE ("MDC"), x=w586) -> (*(type *) &x=w584:bool)
        "B2O" <- w584
        n584 = Not(x=w584) -> (.not. x?=→"B2C":bool)
      }
      frame "B3" {
        n585 = Type Cast(type=TRUE ("MDC"), x=w591) -> (*(type *) &x=w588:bool)
        "B3O" <- w588
        n586 = Not(x=w588) -> (.not. x?=→"B3C":bool)
      }
      frame "MB" {
        n587 = Type Cast(type=TRUE ("MDC"), x=w594) -> (*(type *) &x=w592:bool)
        "MBO" <- w592
        n588 = Not(x=w592) -> (.not. x?=→"MBC":bool)
      }
      frame "B1" {
        n589 = Type Cast(type=TRUE ("MDC"), x=w598) -> (*(type *) &x=w596:bool)
        "B1O" <- w596
        n590 = Not(x=w596) -> (.not. x?=→"B1C":bool)
      }
      frame "TB" {
        n591 = Type Cast(type=TRUE ("MDC"), x=w602) -> (*(type *) &x=w600:bool)
        "TBO" <- w600
        n592 = Not(x=w600) -> (.not. x?=→"TBC":bool)
      }
    }
  }
  n593 = TCP Close Connection "TCP Close \nConnection"(connection ID=w48, error in (no error)=w49) -> (error out=w50:errorcluster)  [unwired: 1 in, 1 out]
  n594 = call <vilib>:"Clear Errors.vi"("error in (no error)"=w50) -> ()  [unwired: 5 in, 2 out]
  n595 = TCP Close Connection "TCP Close \nConnection"(connection ID=w58, error in (no error)=w56) -> (error out=w63:errorcluster)  [unwired: 1 in, 1 out]
  n596 = call <vilib>:"Clear Errors.vi"("error in (no error)"=w63) -> ()  [unwired: 5 in, 2 out]
  n597 = while "Door Automatically Open" {
    stop <- "Door Stop" stop-if-true
    n598 = local read "Open Door"() -> (w605:bool)
    n599 = event shown="[0] \"MDC\": Mouse Enter" {
      selector: _ -> [_ _ _ _ _ _ _ _ _ _ _ _ _ _ _ _]
      dyn-events: _ -> [_ _ _ _ _ _ _ _ _ _ _ _ _ _ _ _]
      timeout: _ -> [_ _ _ _ _ _ _ _ _ _ _ _ _ _ _ _]
      tunnel: w605 -> [w606 w609 w612 w615 w618 w621 w624 w627 w630 w633 w636 w639 w642 w645 w648 w650]
      event "MDC": Mouse Enter {
        n600 = event-data() -> ()  [unwired: 1 in, 1 out]
        n601 = case shown="True" w606 {
          frame False {
          }
          frame True {
            n602 = local write "MDO"(TRUE ("MDO")) -> ()
            n603 = local write "MDC"(FALSE ("MDC")) -> ()
          }
        }
      }
      event "MDC": Mouse Leave {
        n604 = event-data() -> ()  [unwired: 1 in, 1 out]
        n605 = case shown="True" w609 {
          frame False {
          }
          frame True {
            n606 = local write "MDO"(FALSE ("MDO")) -> ()
            n607 = local write "MDC"(TRUE ("MDC")) -> ()
          }
        }
      }
      event "B2C": Mouse Enter {
        n608 = event-data() -> ()  [unwired: 1 in, 1 out]
        n609 = case shown="False" w612 {
          frame False {
          }
          frame True {
            n610 = local write "B2O"(TRUE ("B2O")) -> ()
            n611 = local write "B2C"(FALSE ("B2C")) -> ()
          }
        }
      }
      event "B2C": Mouse Leave {
        n612 = event-data() -> ()  [unwired: 1 in, 1 out]
        n613 = case shown="True" w615 {
          frame False {
          }
          frame True {
            n614 = local write "B2O"(FALSE ("B2O")) -> ()
            n615 = local write "B2C"(TRUE ("B2C")) -> ()
          }
        }
      }
      event "B3C": Mouse Enter {
        n616 = event-data() -> ()  [unwired: 1 in, 1 out]
        n617 = case shown="False" w618 {
          frame False {
          }
          frame True {
            n618 = local write "B3O"(TRUE ("B3O")) -> ()
            n619 = local write "B3C"(FALSE ("B3C")) -> ()
          }
        }
      }
      event "B3C": Mouse Leave {
        n620 = event-data() -> ()  [unwired: 1 in, 1 out]
        n621 = case shown="False" w621 {
          frame False {
          }
          frame True {
            n622 = local write "B3O"(FALSE ("B3O")) -> ()
            n623 = local write "B3C"(TRUE ("B3C")) -> ()
          }
        }
      }
      event "TBC": Mouse Enter {
        n624 = event-data() -> ()  [unwired: 1 in, 1 out]
        n625 = case shown="True" w624 {
          frame False {
          }
          frame True {
            n626 = local write "TBO"(TRUE ("TBO")) -> ()
            n627 = local write "TBC"(FALSE ("TBC")) -> ()
          }
        }
      }
      event "TBC": Mouse Leave {
        n628 = event-data() -> ()  [unwired: 1 in, 1 out]
        n629 = case shown="True" w627 {
          frame False {
          }
          frame True {
            n630 = local write "TBO"(FALSE ("TBO")) -> ()
            n631 = local write "TBC"(TRUE ("TBC")) -> ()
          }
        }
      }
      event "SLC": Mouse Enter {
        n632 = event-data() -> ()  [unwired: 1 in, 1 out]
        n633 = case shown="True" w630 {
          frame False {
          }
          frame True {
            n634 = local write "SLO"(TRUE ("SLO")) -> ()
            n635 = local write "SLC"(FALSE ("SLC")) -> ()
          }
        }
      }
      event "SLC": Mouse Leave {
        n636 = event-data() -> ()  [unwired: 1 in, 1 out]
        n637 = case shown="True" w633 {
          frame False {
          }
          frame True {
            n638 = local write "SLO"(FALSE ("SLO")) -> ()
            n639 = local write "SLC"(TRUE ("SLC")) -> ()
          }
        }
      }
      event "MBC": Mouse Enter {
        n640 = event-data() -> ()  [unwired: 1 in, 1 out]
        n641 = case shown="True" w636 {
          frame False {
          }
          frame True {
            n642 = local write "MBO"(TRUE ("MBO")) -> ()
            n643 = local write "MBC"(FALSE ("MBC")) -> ()
          }
        }
      }
      event "MBC": Mouse Leave {
        n644 = event-data() -> ()  [unwired: 1 in, 1 out]
        n645 = case shown="True" w639 {
          frame False {
          }
          frame True {
            n646 = local write "MBO"(FALSE ("MBO")) -> ()
            n647 = local write "MBC"(TRUE ("MBC")) -> ()
          }
        }
      }
      event "B1C": Mouse Enter {
        n648 = event-data() -> ()  [unwired: 1 in, 1 out]
        n649 = case shown="False" w642 {
          frame False {
          }
          frame True {
            n650 = local write "B1O"(TRUE ("B1O")) -> ()
            n651 = local write "B1C"(FALSE ("B1C")) -> ()
          }
        }
      }
      event "B1C": Mouse Leave {
        n652 = event-data() -> ()  [unwired: 1 in, 1 out]
        n653 = case shown="True" w645 {
          frame False {
          }
          frame True {
            n654 = local write "B1O"(FALSE ("B1O")) -> ()
            n655 = local write "B1C"(TRUE ("B1C")) -> ()
          }
        }
      }
      event "LA": Mouse Enter {
        n656 = event-data() -> ()  [unwired: 1 in, 1 out]
        n657 = case shown="False" w648 {
          frame False {
          }
          frame True {
            n658 = local write "LA"(TRUE ("LAO")) -> ()
          }
        }
      }
      event "LA": Mouse Leave {
        n659 = event-data() -> ()  [unwired: 1 in, 1 out]
        n660 = case shown="True" w650 {
          frame False {
          }
          frame True {
            n661 = local write "LA"(FALSE ("LAO")) -> ()
          }
        }
      }
    }
  }
  n662 = call <vilib>:"TCP Listen.vi"("timeout ms (wait forever: -1)"=-1 ("timeout ms (60000)"), "port"=u16 51114 ("remote port or service name"), "service name"="localhost") -> ("error out"=w28:errorcluster, "connection ID"=w29:refnum<k5>)  [unwired: 4 in, 3 out]
  n663 = local write "KCW2"(w3) -> ()
  n664 = local write "KCW1"(w3) -> ()
  n665 = local write "B3W2"(w3) -> ()
  n666 = local write "B3W1"(w3) -> ()
  n667 = local write "B2W2"(w3) -> ()
  n668 = local write "B2W1"(w3) -> ()
  n669 = local write "MBW"(w3) -> ()
  n670 = local write "LAW"(w3) -> ()
  n671 = while "Curtain" {
    tunnel: w28 -> [w658]
    tunnel: w29 -> [w657]
    tunnel: [w656] -> w31
    tunnel: [w655] -> w32
    stop <- FALSE stop-if-true
    n672 = TCP Read "TCP Read\nReceiving\nData"(connection ID=w657, bytes to read=4, error in (no error)=w658) -> (connection ID out=w661:refnum<k5>, data out=w664:string, error out=w660:errorcluster)  [unwired: 2 in]
    n673 = Type Cast(type=1 ("bytes to read"), x=w664) -> (*(type *) &x=w662:i32)
    n674 = TCP Read "TCP Read\nReceiving\nData"(connection ID=w661, bytes to read=w662, error in (no error)=w660) -> (connection ID out=w655:refnum<k5>, data out=w659:string, error out=w656:errorcluster)  [unwired: 2 in]
    n675 = Search/Split String "Search/\nSplit String"(string=w659, offset (0)=2) -> (substring before match=w653:string, match + rest of string=w652:string)  [unwired: 1 in, 1 out]
    n676 = case shown="\"00\"" w653 {
      tunnel: w652 -> [_ w669 w672 w675 w678 w681 w684 w687 w690]
      frame "False", Default {
      }
      frame "00" {
        n677 = Decimal String To Number "Decimal String \nTo Number"(string=w669) -> (number=w668:i32)  [unwired: 2 in, 1 out]
        n678 = To Double Precision Float(number=w668) -> (double precision float=→"LAW":dbl)
      }
      frame "01" {
        n679 = Decimal String To Number "Decimal String \nTo Number"(string=w672) -> (number=w671:i32)  [unwired: 2 in, 1 out]
        n680 = To Double Precision Float(number=w671) -> (double precision float=→"MBW":dbl)
      }
      frame "02" {
        n681 = Decimal String To Number "Decimal String \nTo Number"(string=w675) -> (number=w674:i32)  [unwired: 2 in, 1 out]
        n682 = To Double Precision Float(number=w674) -> (double precision float=→"B2W1":dbl)
      }
      frame "03" {
        n683 = Decimal String To Number "Decimal String \nTo Number"(string=w678) -> (number=w677:i32)  [unwired: 2 in, 1 out]
        n684 = To Double Precision Float(number=w677) -> (double precision float=→"B2W2":dbl)
      }
      frame "04" {
        n685 = Decimal String To Number "Decimal String \nTo Number"(string=w681) -> (number=w680:i32)  [unwired: 2 in, 1 out]
        n686 = To Double Precision Float(number=w680) -> (double precision float=→"B3W1":dbl)
      }
      frame "05" {
        n687 = Decimal String To Number "Decimal String \nTo Number"(string=w684) -> (number=w683:i32)  [unwired: 2 in, 1 out]
        n688 = To Double Precision Float(number=w683) -> (double precision float=→"B3W2":dbl)
      }
      frame "06" {
        n689 = Decimal String To Number "Decimal String \nTo Number"(string=w687) -> (number=w686:i32)  [unwired: 2 in, 1 out]
        n690 = To Double Precision Float(number=w686) -> (double precision float=→"KCW1":dbl)
      }
      frame "07" {
        n691 = Decimal String To Number "Decimal String \nTo Number"(string=w690) -> (number=w689:i32)  [unwired: 2 in, 1 out]
        n692 = To Double Precision Float(number=w689) -> (double precision float=→"KCW2":dbl)
      }
    }
  }
  n693 = while "Fire Alarm System" {
    stop <- FALSE stop-if-true
    n694 = flat-sequence {
      frame #0 {
        n695 = while "Fire Alarm System" {
          stop <- w692 stop-if-true
          n696 = local read "Temperature"() -> (w694:u8)
          n697 = In Range and Coerce(upper limit=u8 100, x=w694, lower limit=u8 50 ("y")) -> (In Range?=w695:bool)  [unwired: 1 out]
          n698 = local write "Fire Alarm"(w695) -> ()
          n699 = case "Fire Alarm System" shown="True" w695 {
            selector: w695 -> [_ w700]
            frame False {
            }
            frame True {
              w697 = TRUE ("B2O")
              w698 = 0.0 ("B2W2")
              n700 = call <vilib>:"Beep.vi"("use system alert? (T)"=w700) -> ()  [unwired: 11 in]
              n701 = local write "LAW"(w698) -> ()
              n702 = local write "MBW"(w698) -> ()
              n703 = local write "B2W1"(w698) -> ()
              n704 = local write "B2W2"(w698) -> ()
              n705 = local write "B3W1"(w698) -> ()
              n706 = local write "B3W2"(w698) -> ()
              n707 = local write "KCW1"(w698) -> ()
              n708 = local write "KCW2"(w698) -> ()
              n709 = local write "MDO"(w697) -> ()
              n710 = local write "SLO"(w697) -> ()
              n711 = local write "B2O"(w697) -> ()
              n712 = local write "B3O"(w697) -> ()
              n713 = local write "MBO"(w697) -> ()
              n714 = local write "B1O"(w697) -> ()
              n715 = local write "TBO"(w697) -> ()
              n716 = local write "LA"(w697) -> ()
              n717 = Not(x=w697) -> (.not. x?=w699:bool)
              n718 = local write "MDC"(w699) -> ()
              n719 = local write "SLC"(w699) -> ()
              n720 = local write "B2C"(w699) -> ()
              n721 = local write "B3C"(w699) -> ()
              n722 = local write "MBC"(w699) -> ()
              n723 = local write "B1C"(w699) -> ()
              n724 = local write "TBC"(w699) -> ()
              n725 = call "Display Message to User"() -> ()  [unwired: 10 in, 2 out]
            }
          }
          n726 = local read "Fire Alarm"() -> (w692:bool)
        }
      }
      frame #1 {
        n727 = local write "Fire Alarm"(FALSE ("ABC")) -> ()
        n728 = local write "Temperature"(u8 49 ("Temperature")) -> ()
      }
    }
  }
  n729 = local write "AC1"(w4) -> ()
  n730 = local write "AC2"(w4) -> ()
  n731 = call <vilib>:"TCP Listen.vi"("timeout ms (wait forever: -1)"=-1 ("timeout ms (60000)"), "port"=u16 51116 ("remote port or service name"), "service name"="localhost") -> ("error out"=w8:errorcluster, "connection ID"=w9:refnum<k5>)  [unwired: 4 in, 3 out]
  n732 = local write "AC3"(w4) -> ()
  n733 = local write "AC4"(w4) -> ()
  n734 = TCP Close Connection "TCP Close \nConnection"(connection ID=w32, error in (no error)=w31) -> (error out=w30:errorcluster)  [unwired: 1 in, 1 out]
  n735 = while "Air-Conditional" {
    tunnel: w8 -> [w709]
    tunnel: w9 -> [w708]
    tunnel: [w707] -> w11
    tunnel: [w706] -> w12
    stop <- FALSE stop-if-true
    n736 = TCP Read "TCP Read\nReceiving\nData"(connection ID=w708, bytes to read=4, error in (no error)=w709) -> (connection ID out=w712:refnum<k5>, data out=w715:string, error out=w711:errorcluster)  [unwired: 2 in]
    n737 = Type Cast(type=1 ("bytes to read"), x=w715) -> (*(type *) &x=w713:i32)
    n738 = TCP Read "TCP Read\nReceiving\nData"(connection ID=w712, bytes to read=w713, error in (no error)=w711) -> (connection ID out=w706:refnum<k5>, data out=w710:string, error out=w707:errorcluster)  [unwired: 2 in]
    n739 = Search/Split String "Search/\nSplit String"(string=w710, offset (0)=3) -> (substring before match=w704:string, match + rest of string=w703:string)  [unwired: 1 in, 1 out]
    n740 = case shown="\"AC4\"" w704 {
      tunnel: w703 -> [_ w718 w721 w724 w727]
      frame "False", Default {
      }
      frame "AC1" {
        n741 = Type Cast(type=TRUE, x=w718) -> (*(type *) &x=→"AC1":bool)
      }
      frame "AC2" {
        n742 = Type Cast(type=TRUE, x=w721) -> (*(type *) &x=→"AC2":bool)
      }
      frame "AC3" {
        n743 = Type Cast(type=TRUE, x=w724) -> (*(type *) &x=→"AC3":bool)
      }
      frame "AC4" {
        n744 = Type Cast(type=TRUE, x=w727) -> (*(type *) &x=→"AC4":bool)
      }
    }
  }
  n745 = call <vilib>:"Clear Errors.vi"("error in (no error)"=w30) -> ()  [unwired: 5 in, 2 out]
  n746 = call <vilib>:"TCP Listen.vi"("timeout ms (wait forever: -1)"=-1 ("timeout ms (60000)"), "port"=u16 51115 ("remote port or service name"), "service name"="localhost") -> ("error out"=w19:errorcluster, "connection ID"=w18:refnum<k5>)  [unwired: 4 in, 3 out]
  n747 = while "Brightness" {
    tunnel: w19 -> [w736]
    tunnel: w18 -> [w735]
    tunnel: [w734] -> w16
    tunnel: [w733] -> w15
    stop <- FALSE stop-if-true
    n748 = TCP Read "TCP Read\nReceiving\nData"(connection ID=w735, bytes to read=4, error in (no error)=w736) -> (connection ID out=w739:refnum<k5>, data out=w742:string, error out=w738:errorcluster)  [unwired: 2 in]
    n749 = Type Cast(type=1 ("bytes to read"), x=w742) -> (*(type *) &x=w740:i32)
    n750 = TCP Read "TCP Read\nReceiving\nData"(connection ID=w739, bytes to read=w740, error in (no error)=w738) -> (connection ID out=w733:refnum<k5>, data out=w737:string, error out=w734:errorcluster)  [unwired: 2 in]
    n751 = Search/Split String "Search/\nSplit String"(string=w737, offset (0)=2) -> (substring before match=w731:string, match + rest of string=w730:string)  [unwired: 1 in, 1 out]
    n752 = case shown="\"01\"" w731 {
      tunnel: w730 -> [_ w747 w750 w753 w756 w759 w762 w765 w768 w771 w774 w777 w780 w783 w786 w789 w792 w795 w798 w801 w804 w807 w810]
      frame "False", Default {
      }
      frame "00" {
        n753 = Decimal String To Number "Decimal String \nTo Number"(string=w747) -> (number=w746:i32)  [unwired: 2 in, 1 out]
        n754 = To Unsigned Byte Integer "To Unsigned\n Byte Integer"(number=w746) -> (unsigned 8bit integer=→"Brightness\nMaster Bedroom \nLight 1":u8)
      }
      frame "01" {
        n755 = Decimal String To Number "Decimal String \nTo Number"(string=w750) -> (number=w749:i32)  [unwired: 2 in, 1 out]
        n756 = To Unsigned Byte Integer "To Unsigned\n Byte Integer"(number=w749) -> (unsigned 8bit integer=→"Brightness\nKitchen \nLight 1":u8)
      }
      frame "02" {
        n757 = Decimal String To Number "Decimal String \nTo Number"(string=w753) -> (number=w752:i32)  [unwired: 2 in, 1 out]
        n758 = To Unsigned Byte Integer "To Unsigned\n Byte Integer"(number=w752) -> (unsigned 8bit integer=→"Brightness\nKitchen \nLight 2":u8)
      }
      frame "03" {
        n759 = Decimal String To Number "Decimal String \nTo Number"(string=w756) -> (number=w755:i32)  [unwired: 2 in, 1 out]
        n760 = To Unsigned Byte Integer "To Unsigned\n Byte Integer"(number=w755) -> (unsigned 8bit integer=→"Brightness\nService Laundry \nLight 1":u8)
      }
      frame "04" {
        n761 = Decimal String To Number "Decimal String \nTo Number"(string=w759) -> (number=w758:i32)  [unwired: 2 in, 1 out]
        n762 = To Unsigned Byte Integer "To Unsigned\n Byte Integer"(number=w758) -> (unsigned 8bit integer=→"Brightness\nService Laundry \nLight 2":u8)
      }
      frame "05" {
        n763 = Decimal String To Number "Decimal String \nTo Number"(string=w762) -> (number=w761:i32)  [unwired: 2 in, 1 out]
        n764 = To Unsigned Byte Integer "To Unsigned\n Byte Integer"(number=w761) -> (unsigned 8bit integer=→"Brightness\nT&B Light":u8)
      }
      frame "06" {
        n765 = Decimal String To Number "Decimal String \nTo Number"(string=w765) -> (number=w764:i32)  [unwired: 2 in, 1 out]
        n766 = To Unsigned Byte Integer "To Unsigned\n Byte Integer"(number=w764) -> (unsigned 8bit integer=→"Brightness\nMaster Bedroom \nLight 2":u8)
      }
      frame "07" {
        n767 = Decimal String To Number "Decimal String \nTo Number"(string=w768) -> (number=w767:i32)  [unwired: 2 in, 1 out]
        n768 = To Unsigned Byte Integer "To Unsigned\n Byte Integer"(number=w767) -> (unsigned 8bit integer=→"Brightness\nMaster Bedroom \nW.I.C. Light":u8)
      }
      frame "08" {
        n769 = Decimal String To Number "Decimal String \nTo Number"(string=w771) -> (number=w770:i32)  [unwired: 2 in, 1 out]
        n770 = To Unsigned Byte Integer "To Unsigned\n Byte Integer"(number=w770) -> (unsigned 8bit integer=→"Brightness\nLiving Area Light 1":u8)
      }
      frame "09" {
        n771 = Decimal String To Number "Decimal String \nTo Number"(string=w774) -> (number=w773:i32)  [unwired: 2 in, 1 out]
        n772 = To Unsigned Byte Integer "To Unsigned\n Byte Integer"(number=w773) -> (unsigned 8bit integer=→"Brightness\nLiving Area Light 2":u8)
      }
      frame "10" {
        n773 = Decimal String To Number "Decimal String \nTo Number"(string=w777) -> (number=w776:i32)  [unwired: 2 in, 1 out]
        n774 = To Unsigned Byte Integer "To Unsigned\n Byte Integer"(number=w776) -> (unsigned 8bit integer=→"Brightness\n Porch Light":u8)
      }
      frame "11" {
        n775 = Decimal String To Number "Decimal String \nTo Number"(string=w780) -> (number=w779:i32)  [unwired: 2 in, 1 out]
        n776 = To Unsigned Byte Integer "To Unsigned\n Byte Integer"(number=w779) -> (unsigned 8bit integer=→"Brightness\nDining Area Light 1":u8)
      }
      frame "12" {
        n777 = Decimal String To Number "Decimal String \nTo Number"(string=w783) -> (number=w782:i32)  [unwired: 2 in, 1 out]
        n778 = To Unsigned Byte Integer "To Unsigned\n Byte Integer"(number=w782) -> (unsigned 8bit integer=→"Brightness\nDining Area Light 2":u8)
      }
      frame "13" {
        n779 = Decimal String To Number "Decimal String \nTo Number"(string=w786) -> (number=w785:i32)  [unwired: 2 in, 1 out]
        n780 = To Unsigned Byte Integer "To Unsigned\n Byte Integer"(number=w785) -> (unsigned 8bit integer=→"Brightness\nLanai Light":u8)
      }
      frame "14" {
        n781 = Decimal String To Number "Decimal String \nTo Number"(string=w789) -> (number=w788:i32)  [unwired: 2 in, 1 out]
        n782 = To Unsigned Byte Integer "To Unsigned\n Byte Integer"(number=w788) -> (unsigned 8bit integer=→"Brightness\nBedroom 2 \nLight 1":u8)
      }
      frame "15" {
        n783 = Decimal String To Number "Decimal String \nTo Number"(string=w792) -> (number=w791:i32)  [unwired: 2 in, 1 out]
        n784 = To Unsigned Byte Integer "To Unsigned\n Byte Integer"(number=w791) -> (unsigned 8bit integer=→"Brightness\nBedroom 2 \nLight 2":u8)
      }
      frame "16" {
        n785 = Decimal String To Number "Decimal String \nTo Number"(string=w795) -> (number=w794:i32)  [unwired: 2 in, 1 out]
        n786 = To Unsigned Byte Integer "To Unsigned\n Byte Integer"(number=w794) -> (unsigned 8bit integer=→"Brightness\nBedroom 2 \nW.I.C. Light":u8)
      }
      frame "17" {
        n787 = Decimal String To Number "Decimal String \nTo Number"(string=w798) -> (number=w797:i32)  [unwired: 2 in, 1 out]
        n788 = To Unsigned Byte Integer "To Unsigned\n Byte Integer"(number=w797) -> (unsigned 8bit integer=→"Brightness\nBedroom 3 \nLight 1":u8)
      }
      frame "18" {
        n789 = Decimal String To Number "Decimal String \nTo Number"(string=w801) -> (number=w800:i32)  [unwired: 2 in, 1 out]
        n790 = To Unsigned Byte Integer "To Unsigned\n Byte Integer"(number=w800) -> (unsigned 8bit integer=→"Brightness\nBedroom 3 \nLight 2":u8)
      }
      frame "19" {
        n791 = Decimal String To Number "Decimal String \nTo Number"(string=w804) -> (number=w803:i32)  [unwired: 2 in, 1 out]
        n792 = To Unsigned Byte Integer "To Unsigned\n Byte Integer"(number=w803) -> (unsigned 8bit integer=→"Brightness\nGarage Light 1":u8)
      }
      frame "20" {
        n793 = Decimal String To Number "Decimal String \nTo Number"(string=w807) -> (number=w806:i32)  [unwired: 2 in, 1 out]
        n794 = To Unsigned Byte Integer "To Unsigned\n Byte Integer"(number=w806) -> (unsigned 8bit integer=→"Brightness\nGarage Light 2":u8)
      }
      frame "21" {
        n795 = Decimal String To Number "Decimal String \nTo Number"(string=w810) -> (number=w809:i32)  [unwired: 2 in, 1 out]
        n796 = To Unsigned Byte Integer "To Unsigned\n Byte Integer"(number=w809) -> (unsigned 8bit integer=→"Brightness\nMaster Bath \nLight":u8)
      }
    }
  }
  n797 = TCP Close Connection "TCP Close \nConnection"(connection ID=w12, error in (no error)=w11) -> (error out=w10:errorcluster)  [unwired: 1 in, 1 out]
  n798 = call <vilib>:"Clear Errors.vi"("error in (no error)"=w10) -> ()  [unwired: 5 in, 2 out]
  n799 = local write "Brightness\nBedroom 2 \nW.I.C. Light"(w13) -> ()
  n800 = local write "Brightness\nMaster Bath \nLight"(w13) -> ()
  n801 = local write "Brightness\nT&B Light"(w13) -> ()
  n802 = local write "Brightness\nService Laundry \nLight 2"(w13) -> ()
  n803 = local write "Brightness\n Porch Light"(w13) -> ()
  n804 = local write "Brightness\nService Laundry \nLight 1"(w13) -> ()
  n805 = local write "Brightness\nLiving Area Light 2"(w13) -> ()
  n806 = local write "Brightness\nLiving Area Light 1"(w13) -> ()
  n807 = local write "Brightness\nKitchen \nLight 2"(w13) -> ()
  n808 = local write "Brightness\nKitchen \nLight 1"(w13) -> ()
  n809 = local write "Brightness\nMaster Bedroom \nW.I.C. Light"(w13) -> ()
  n810 = local write "Brightness\nMaster Bedroom \nLight 1"(w13) -> ()
  n811 = local write "Brightness\nDining Area Light 2"(w13) -> ()
  n812 = local write "Brightness\nLanai Light"(w13) -> ()
  n813 = local write "Brightness\nBedroom 2 \nLight 2"(w13) -> ()
  n814 = local write "Brightness\nBedroom 2 \nLight 1"(w13) -> ()
  n815 = local write "Brightness\nGarage Light 2"(w13) -> ()
  n816 = local write "Brightness\nGarage Light 1"(w13) -> ()
  n817 = local write "Brightness\nBedroom 3 \nLight 2"(w13) -> ()
  n818 = local write "Brightness\nBedroom 3 \nLight 1"(w13) -> ()
  n819 = local write "Brightness\nMaster Bedroom \nLight 2"(w13) -> ()
  n820 = local write "Brightness\nDining Area Light 1"(w13) -> ()
  n821 = TCP Close Connection "TCP Close \nConnection"(connection ID=w15, error in (no error)=w16) -> (error out=w17:errorcluster)  [unwired: 1 in, 1 out]
  n822 = call <vilib>:"Clear Errors.vi"("error in (no error)"=w17) -> ()  [unwired: 5 in, 2 out]
  n823 = while "Brightness" {
    stop <- FALSE stop-if-true
    n824 = local read "Temperature"() -> (w819:u8)
    n825 = In Range and Coerce(upper limit=51, x=w819, lower limit=30 ("y")) -> (In Range?=w818:bool)  [unwired: 1 out]
    n826 = case shown="True" w818 {
      frame False {
      }
      frame True {
        w1218 = i8 0 ("hi")
        w1259 = i8 0 ("hi")
        w1260 = i8 0 ("hi")
        w1271 = i8 0 ("hi")
        w1272 = i8 0 ("hi")
        w1283 = i8 0 ("hi")
        w1248 = i8 0 ("hi")
        w1247 = i8 0 ("hi")
        w1236 = i8 0 ("hi")
        w1235 = i8 0 ("hi")
        w1224 = i8 0 ("hi")
        w1308 = i8 0 ("hi")
        w1307 = i8 0 ("hi")
        w1296 = i8 0 ("hi")
        w1295 = i8 0 ("hi")
        w1284 = i8 0 ("hi")
        w1319 = i8 0 ("hi")
        w1320 = i8 0 ("hi")
        w1331 = i8 0 ("hi")
        w1332 = i8 0 ("hi")
        w1343 = i8 0 ("hi")
        w1344 = i8 0 ("hi")
        n827 = local read "Brightness\nMaster Bedroom \nLight 1"() -> (w1346:u8)
        n828 = local read "Brightness\nDining Area Light 2"() -> (w1197:u8)
        n829 = local read "Brightness\nLanai Light"() -> (w1198:u8)
        n830 = local read "Brightness\nBedroom 2 \nLight 1"() -> (w1199:u8)
        n831 = local read "Brightness\nBedroom 2 \nLight 2"() -> (w1200:u8)
        n832 = local read "Brightness\nGarage Light 2"() -> (w1201:u8)
        n833 = local read "Brightness\nGarage Light 1"() -> (w1202:u8)
        n834 = local read "Brightness\nBedroom 3 \nLight 2"() -> (w1203:u8)
        n835 = local read "Brightness\nBedroom 3 \nLight 1"() -> (w1204:u8)
        n836 = local read "Brightness\nBedroom 2 \nW.I.C. Light"() -> (w1205:u8)
        n837 = local read "Brightness\nMaster Bath \nLight"() -> (w1207:u8)
        n838 = local read "Brightness\nT&B Light"() -> (w1206:u8)
        n839 = local read "Brightness\nService Laundry \nLight 2"() -> (w1208:u8)
        n840 = local read "Brightness\nService Laundry \nLight 1"() -> (w1209:u8)
        n841 = local read "Brightness\nKitchen \nLight 2"() -> (w1210:u8)
        n842 = local read "Brightness\nKitchen \nLight 1"() -> (w1211:u8)
        n843 = local read "Brightness\n Porch Light"() -> (w1212:u8)
        n844 = local read "Brightness\nLiving Area Light 2"() -> (w1213:u8)
        n845 = local read "Brightness\nLiving Area Light 1"() -> (w1214:u8)
        n846 = local read "Brightness\nMaster Bedroom \nW.I.C. Light"() -> (w1215:u8)
        n847 = local read "Brightness\nMaster Bedroom \nLight 2"() -> (w1216:u8)
        n848 = local read "Brightness\nDining Area Light 1"() -> (w1217:u8)
        n849 = Join Numbers(hi=w1332, lo=w1198) -> ((hi.lo)=w1336:u16)
        n850 = Join Numbers(hi=w1332, lo=w1332) -> ((hi.lo)=w1335:u16)
        n851 = Join Numbers(hi=w1344, lo=w1346) -> ((hi.lo)=w1349:u16)
        n852 = Join Numbers(hi=w1344, lo=w1344) -> ((hi.lo)=w1348:u16)
        n853 = Join Numbers(hi=w1343, lo=w1197) -> ((hi.lo)=w1339:u16)
        n854 = Join Numbers(hi=w1343, lo=w1343) -> ((hi.lo)=w1340:u16)
        n855 = Join Numbers(hi=w1331, lo=w1199) -> ((hi.lo)=w1327:u16)
        n856 = Join Numbers(hi=w1331, lo=w1331) -> ((hi.lo)=w1328:u16)
        n857 = Join Numbers(hi=w1295, lo=w1203) -> ((hi.lo)=w1291:u16)
        n858 = Join Numbers(hi=w1295, lo=w1295) -> ((hi.lo)=w1292:u16)
        n859 = Join Numbers(hi=w1320, lo=w1200) -> ((hi.lo)=w1324:u16)
        n860 = Join Numbers(hi=w1320, lo=w1320) -> ((hi.lo)=w1323:u16)
        n861 = Join Numbers(hi=w1319, lo=w1201) -> ((hi.lo)=w1315:u16)
        n862 = Join Numbers(hi=w1319, lo=w1319) -> ((hi.lo)=w1316:u16)
        n863 = Join Numbers(hi=w1284, lo=w1202) -> ((hi.lo)=w1288:u16)
        n864 = Join Numbers(hi=w1284, lo=w1284) -> ((hi.lo)=w1287:u16)
        n865 = Join Numbers(hi=w1296, lo=w1204) -> ((hi.lo)=w1300:u16)
        n866 = Join Numbers(hi=w1296, lo=w1296) -> ((hi.lo)=w1299:u16)
        n867 = Join Numbers(hi=w1235, lo=w1208) -> ((hi.lo)=w1231:u16)
        n868 = Join Numbers(hi=w1235, lo=w1235) -> ((hi.lo)=w1232:u16)
        n869 = Join Numbers(hi=w1307, lo=w1205) -> ((hi.lo)=w1303:u16)
        n870 = Join Numbers(hi=w1307, lo=w1307) -> ((hi.lo)=w1304:u16)
        n871 = Join Numbers(hi=w1308, lo=w1207) -> ((hi.lo)=w1312:u16)
        n872 = Join Numbers(hi=w1308, lo=w1308) -> ((hi.lo)=w1311:u16)
        n873 = Join Numbers(hi=w1224, lo=w1206) -> ((hi.lo)=w1228:u16)
        n874 = Join Numbers(hi=w1224, lo=w1224) -> ((hi.lo)=w1227:u16)
        n875 = Join Numbers(hi=w1236, lo=w1209) -> ((hi.lo)=w1240:u16)
        n876 = Join Numbers(hi=w1236, lo=w1236) -> ((hi.lo)=w1239:u16)
        n877 = Join Numbers(hi=w1272, lo=w1213) -> ((hi.lo)=w1276:u16)
        n878 = Join Numbers(hi=w1272, lo=w1272) -> ((hi.lo)=w1275:u16)
        n879 = Join Numbers(hi=w1247, lo=w1210) -> ((hi.lo)=w1243:u16)
        n880 = Join Numbers(hi=w1247, lo=w1247) -> ((hi.lo)=w1244:u16)
        n881 = Join Numbers(hi=w1248, lo=w1211) -> ((hi.lo)=w1252:u16)
        n882 = Join Numbers(hi=w1248, lo=w1248) -> ((hi.lo)=w1251:u16)
        n883 = Join Numbers(hi=w1283, lo=w1212) -> ((hi.lo)=w1279:u16)
        n884 = Join Numbers(hi=w1283, lo=w1283) -> ((hi.lo)=w1280:u16)
        n885 = Join Numbers(hi=w1271, lo=w1214) -> ((hi.lo)=w1267:u16)
        n886 = Join Numbers(hi=w1271, lo=w1271) -> ((hi.lo)=w1268:u16)
        n887 = Join Numbers(hi=w1260, lo=w1215) -> ((hi.lo)=w1264:u16)
        n888 = Join Numbers(hi=w1260, lo=w1260) -> ((hi.lo)=w1263:u16)
        n889 = Join Numbers(hi=w1259, lo=w1216) -> ((hi.lo)=w1255:u16)
        n890 = Join Numbers(hi=w1259, lo=w1259) -> ((hi.lo)=w1256:u16)
        n891 = Join Numbers(hi=w1336, lo=w1335) -> ((hi.lo)=w1334:u32)
        n892 = Join Numbers(hi=w1218, lo=w1217) -> ((hi.lo)=w1222:u16)
        n893 = Join Numbers(hi=w1218, lo=w1218) -> ((hi.lo)=w1221:u16)
        n894 = Join Numbers(hi=w1349, lo=w1348) -> ((hi.lo)=w1347:u32)
        n895 = Join Numbers(hi=w1339, lo=w1340) -> ((hi.lo)=w1341:u32)
        n896 = Join Numbers(hi=w1327, lo=w1328) -> ((hi.lo)=w1329:u32)
        n897 = Join Numbers(hi=w1291, lo=w1292) -> ((hi.lo)=w1293:u32)
        n898 = Join Numbers(hi=w1324, lo=w1323) -> ((hi.lo)=w1322:u32)
        n899 = Join Numbers(hi=w1315, lo=w1316) -> ((hi.lo)=w1317:u32)
        n900 = Join Numbers(hi=w1288, lo=w1287) -> ((hi.lo)=w1286:u32)
        n901 = Join Numbers(hi=w1300, lo=w1299) -> ((hi.lo)=w1298:u32)
        n902 = Join Numbers(hi=w1231, lo=w1232) -> ((hi.lo)=w1233:u32)
        n903 = Join Numbers(hi=w1303, lo=w1304) -> ((hi.lo)=w1305:u32)
        n904 = Join Numbers(hi=w1312, lo=w1311) -> ((hi.lo)=w1310:u32)
        n905 = Join Numbers(hi=w1228, lo=w1227) -> ((hi.lo)=w1226:u32)
        n906 = Join Numbers(hi=w1240, lo=w1239) -> ((hi.lo)=w1238:u32)
        n907 = Join Numbers(hi=w1276, lo=w1275) -> ((hi.lo)=w1274:u32)
        n908 = Join Numbers(hi=w1243, lo=w1244) -> ((hi.lo)=w1245:u32)
        n909 = Join Numbers(hi=w1252, lo=w1251) -> ((hi.lo)=w1250:u32)
        n910 = Join Numbers(hi=w1279, lo=w1280) -> ((hi.lo)=w1281:u32)
        n911 = Join Numbers(hi=w1267, lo=w1268) -> ((hi.lo)=w1269:u32)
        n912 = Join Numbers(hi=w1264, lo=w1263) -> ((hi.lo)=w1262:u32)
        n913 = Join Numbers(hi=w1255, lo=w1256) -> ((hi.lo)=w1257:u32)
        n914 = Join Numbers(hi=w1222, lo=w1221) -> ((hi.lo)=w1220:u32)
        n915 = Bundle(w1334, w1334) -> (w1337:cluster{u32, u32})  [unwired: 1 in]
        n916 = Bundle(w1347, w1347) -> (w1350:cluster{u32, u32})  [unwired: 1 in]
        n917 = Bundle(w1341, w1341) -> (w1338:cluster{u32, u32})  [unwired: 1 in]
        n918 = Bundle(w1329, w1329) -> (w1326:cluster{u32, u32})  [unwired: 1 in]
        n919 = Bundle(w1293, w1293) -> (w1290:cluster{u32, u32})  [unwired: 1 in]
        n920 = Bundle(w1322, w1322) -> (w1325:cluster{u32, u32})  [unwired: 1 in]
        n921 = Bundle(w1317, w1317) -> (w1314:cluster{u32, u32})  [unwired: 1 in]
        n922 = Bundle(w1286, w1286) -> (w1289:cluster{u32, u32})  [unwired: 1 in]
        n923 = Bundle(w1298, w1298) -> (w1301:cluster{u32, u32})  [unwired: 1 in]
        n924 = Bundle(w1233, w1233) -> (w1230:cluster{u32, u32})  [unwired: 1 in]
        n925 = Bundle(w1305, w1305) -> (w1302:cluster{u32, u32})  [unwired: 1 in]
        n926 = Bundle(w1310, w1310) -> (w1313:cluster{u32, u32})  [unwired: 1 in]
        n927 = Bundle(w1226, w1226) -> (w1229:cluster{u32, u32})  [unwired: 1 in]
        n928 = Bundle(w1238, w1238) -> (w1241:cluster{u32, u32})  [unwired: 1 in]
        n929 = Bundle(w1274, w1274) -> (w1277:cluster{u32, u32})  [unwired: 1 in]
        n930 = Bundle(w1245, w1245) -> (w1242:cluster{u32, u32})  [unwired: 1 in]
        n931 = Bundle(w1250, w1250) -> (w1253:cluster{u32, u32})  [unwired: 1 in]
        n932 = Bundle(w1281, w1281) -> (w1278:cluster{u32, u32})  [unwired: 1 in]
        n933 = Bundle(w1269, w1269) -> (w1266:cluster{u32, u32})  [unwired: 1 in]
        n934 = Bundle(w1262, w1262) -> (w1265:cluster{u32, u32})  [unwired: 1 in]
        n935 = Bundle(w1257, w1257) -> (w1254:cluster{u32, u32})  [unwired: 1 in]
        n936 = Bundle(w1220, w1220) -> (w1223:cluster{u32, u32})  [unwired: 1 in]
        n937 = Build Array "Build Array"(cluster{u32, u32} {0, 0} ("element"), w1337) -> (w1176:cluster{u32, u32}[])
        n938 = Build Array "Build Array"(cluster{u32, u32} {0, 0} ("element"), w1350) -> (w1196:cluster{u32, u32}[])
        n939 = Build Array "Build Array"(cluster{u32, u32} {0, 0} ("element"), w1338) -> (w1175:cluster{u32, u32}[])
        n940 = Build Array "Build Array"(cluster{u32, u32} {0, 0} ("element"), w1326) -> (w1177:cluster{u32, u32}[])
        n941 = Build Array "Build Array"(cluster{u32, u32} {0, 0} ("element"), w1290) -> (w1181:cluster{u32, u32}[])
        n942 = Build Array "Build Array"(cluster{u32, u32} {0, 0} ("element"), w1325) -> (w1178:cluster{u32, u32}[])
        n943 = Build Array "Build Array"(cluster{u32, u32} {0, 0} ("element"), w1314) -> (w1179:cluster{u32, u32}[])
        n944 = Build Array "Build Array"(cluster{u32, u32} {0, 0} ("element"), w1289) -> (w1180:cluster{u32, u32}[])
        n945 = Build Array "Build Array"(cluster{u32, u32} {0, 0} ("element"), w1301) -> (w1182:cluster{u32, u32}[])
        n946 = Build Array "Build Array"(cluster{u32, u32} {0, 0} ("element"), w1230) -> (w1186:cluster{u32, u32}[])
        n947 = Build Array "Build Array"(cluster{u32, u32} {0, 0} ("element"), w1302) -> (w1183:cluster{u32, u32}[])
        n948 = Build Array "Build Array"(cluster{u32, u32} {0, 0} ("element"), w1313) -> (w1184:cluster{u32, u32}[])
        n949 = Build Array "Build Array"(cluster{u32, u32} {0, 0} ("element"), w1229) -> (w1185:cluster{u32, u32}[])
        n950 = Build Array "Build Array"(cluster{u32, u32} {0, 0} ("element"), w1241) -> (w1187:cluster{u32, u32}[])
        n951 = Build Array "Build Array"(cluster{u32, u32} {0, 0} ("element"), w1277) -> (w1191:cluster{u32, u32}[])
        n952 = Build Array "Build Array"(cluster{u32, u32} {0, 0} ("element"), w1242) -> (w1188:cluster{u32, u32}[])
        n953 = Build Array "Build Array"(cluster{u32, u32} {0, 0} ("element"), w1253) -> (w1189:cluster{u32, u32}[])
        n954 = Build Array "Build Array"(cluster{u32, u32} {0, 0} ("element"), w1278) -> (w1190:cluster{u32, u32}[])
        n955 = Build Array "Build Array"(cluster{u32, u32} {0, 0} ("element"), w1266) -> (w1192:cluster{u32, u32}[])
        n956 = Build Array "Build Array"(cluster{u32, u32} {0, 0} ("element"), w1265) -> (w1193:cluster{u32, u32}[])
        n957 = Build Array "Build Array"(cluster{u32, u32} {0, 0} ("element"), w1254) -> (w1194:cluster{u32, u32}[])
        n958 = Build Array "Build Array"(cluster{u32, u32} {0, 0} ("element"), w1223) -> (w1195:cluster{u32, u32}[])
        n959 = property on="KL1" class="Bool (strict)"("Colors [4]"=w1189) -> ()  [unwired: 2 in, 2 out]
        n960 = property on="MBL1" class="Bool (strict)"("Colors [4]"=w1196) -> ()  [unwired: 2 in, 2 out]
        n961 = property on="DAL2" class="Bool (strict)"("Colors [4]"=w1175) -> ()  [unwired: 2 in, 2 out]
        n962 = property on="LL" class="Bool (strict)"("Colors [4]"=w1176) -> ()  [unwired: 2 in, 2 out]
        n963 = property on="B2L2" class="Bool (strict)"("Colors [4]"=w1178) -> ()  [unwired: 2 in, 2 out]
        n964 = property on="GL2" class="Bool (strict)"("Colors [4]"=w1179) -> ()  [unwired: 2 in, 2 out]
        n965 = property on="GL1" class="Bool (strict)"("Colors [4]"=w1180) -> ()  [unwired: 2 in, 2 out]
        n966 = property on="B3L2" class="Bool (strict)"("Colors [4]"=w1181) -> ()  [unwired: 2 in, 2 out]
        n967 = property on="B3L1" class="Bool (strict)"("Colors [4]"=w1182) -> ()  [unwired: 2 in, 2 out]
        n968 = property on="B2WICL" class="Bool (strict)"("Colors [4]"=w1183) -> ()  [unwired: 2 in, 2 out]
        n969 = property on="MBL" class="Bool (strict)"("Colors [4]"=w1184) -> ()  [unwired: 2 in, 2 out]
        n970 = property on="TBL" class="Bool (strict)"("Colors [4]"=w1185) -> ()  [unwired: 2 in, 2 out]
        n971 = property on="SLL2" class="Bool (strict)"("Colors [4]"=w1186) -> ()  [unwired: 2 in, 2 out]
        n972 = property on="SLL1" class="Bool (strict)"("Colors [4]"=w1187) -> ()  [unwired: 2 in, 2 out]
        n973 = property on="KL2" class="Bool (strict)"("Colors [4]"=w1188) -> ()  [unwired: 2 in, 2 out]
        n974 = property on="PL" class="Bool (strict)"("Colors [4]"=w1190) -> ()  [unwired: 2 in, 2 out]
        n975 = property on="LAL2" class="Bool (strict)"("Colors [4]"=w1191) -> ()  [unwired: 2 in, 2 out]
        n976 = property on="LAL1" class="Bool (strict)"("Colors [4]"=w1192) -> ()  [unwired: 2 in, 2 out]
        n977 = property on="MBWICL" class="Bool (strict)"("Colors [4]"=w1193) -> ()  [unwired: 2 in, 2 out]
        n978 = property on="MBL2" class="Bool (strict)"("Colors [4]"=w1194) -> ()  [unwired: 2 in, 2 out]
        n979 = property on="DAL1" class="Bool (strict)"("Colors [4]"=w1195) -> ()  [unwired: 2 in, 2 out]
        n980 = property on="B2L1" class="Bool (strict)"("Colors [4]"=w1177) -> ()  [unwired: 2 in, 2 out]
      }
    }
    n981 = local read "Temperature"() -> (w815:u8)
    n982 = Less?(x=w815, y=u8 10) -> (x < y?=w817:bool)
    n983 = case shown="False" w817 {
      frame False {
      }
      frame True {
        w1047 = i8 0 ("hi")
        w1048 = i8 0 ("hi")
        w1059 = i8 0 ("hi")
        w1060 = i8 0 ("hi")
        w1071 = i8 0 ("hi")
        w1072 = i8 0 ("hi")
        w1083 = i8 0 ("hi")
        w1084 = i8 0 ("hi")
        w1095 = i8 0 ("hi")
        w1096 = i8 0 ("hi")
        w1107 = i8 0 ("hi")
        w1108 = i8 0 ("hi")
        w1119 = i8 0 ("hi")
        w1120 = i8 0 ("hi")
        w1131 = i8 0 ("hi")
        w1132 = i8 0 ("hi")
        w1143 = i8 0 ("hi")
        w1144 = i8 0 ("hi")
        w1155 = i8 0 ("hi")
        w1156 = i8 0 ("hi")
        w1167 = i8 0 ("hi")
        w1168 = i8 0 ("hi")
        n984 = local read "Brightness\nMaster Bath \nLight"() -> (w1011:u8)
        n985 = local read "Brightness\nBedroom 2 \nW.I.C. Light"() -> (w1012:u8)
        n986 = local read "Brightness\nBedroom 2 \nLight 1"() -> (w1018:u8)
        n987 = local read "Brightness\nGarage Light 2"() -> (w1016:u8)
        n988 = local read "Brightness\nBedroom 3 \nLight 2"() -> (w1014:u8)
        n989 = local read "Brightness\nT&B Light"() -> (w1010:u8)
        n990 = local read "Brightness\nBedroom 3 \nLight 1"() -> (w1013:u8)
        n991 = local read "Brightness\nService Laundry \nLight 1"() -> (w1008:u8)
        n992 = local read "Brightness\nBedroom 2 \nLight 2"() -> (w1017:u8)
        n993 = local read "Brightness\nGarage Light 1"() -> (w1015:u8)
        n994 = local read "Brightness\nService Laundry \nLight 2"() -> (w1009:u8)
        n995 = local read "Brightness\nKitchen \nLight 2"() -> (w1007:u8)
        n996 = local read "Brightness\nLiving Area Light 1"() -> (w1003:u8)
        n997 = local read "Brightness\nMaster Bedroom \nLight 1"() -> (w1170:u8)
        n998 = local read "Brightness\nDining Area Light 2"() -> (w1020:u8)
        n999 = local read "Brightness\nLanai Light"() -> (w1019:u8)
        n1000 = local read "Brightness\nLiving Area Light 2"() -> (w1004:u8)
        n1001 = local read "Brightness\nKitchen \nLight 1"() -> (w1006:u8)
        n1002 = local read "Brightness\n Porch Light"() -> (w1005:u8)
        n1003 = local read "Brightness\nMaster Bedroom \nW.I.C. Light"() -> (w1002:u8)
        n1004 = local read "Brightness\nMaster Bedroom \nLight 2"() -> (w1001:u8)
        n1005 = local read "Brightness\nDining Area Light 1"() -> (w1000:u8)
        n1006 = Join Numbers(hi=w1168, lo=w1168) -> ((hi.lo)=w1174:u16)
        n1007 = Join Numbers(hi=w1170, lo=w1168) -> ((hi.lo)=w1173:u16)
        n1008 = Join Numbers(hi=w1167, lo=w1167) -> ((hi.lo)=w1162:u16)
        n1009 = Join Numbers(hi=w1020, lo=w1167) -> ((hi.lo)=w1163:u16)
        n1010 = Join Numbers(hi=w1156, lo=w1156) -> ((hi.lo)=w1161:u16)
        n1011 = Join Numbers(hi=w1019, lo=w1156) -> ((hi.lo)=w1160:u16)
        n1012 = Join Numbers(hi=w1155, lo=w1155) -> ((hi.lo)=w1150:u16)
        n1013 = Join Numbers(hi=w1018, lo=w1155) -> ((hi.lo)=w1151:u16)
        n1014 = Join Numbers(hi=w1144, lo=w1144) -> ((hi.lo)=w1149:u16)
        n1015 = Join Numbers(hi=w1017, lo=w1144) -> ((hi.lo)=w1148:u16)
        n1016 = Join Numbers(hi=w1143, lo=w1143) -> ((hi.lo)=w1138:u16)
        n1017 = Join Numbers(hi=w1016, lo=w1143) -> ((hi.lo)=w1139:u16)
        n1018 = Join Numbers(hi=w1174, lo=w1173) -> ((hi.lo)=w1172:u32)
        n1019 = Join Numbers(hi=w1132, lo=w1132) -> ((hi.lo)=w1137:u16)
        n1020 = Join Numbers(hi=w1015, lo=w1132) -> ((hi.lo)=w1136:u16)
        n1021 = Join Numbers(hi=w1131, lo=w1131) -> ((hi.lo)=w1126:u16)
        n1022 = Join Numbers(hi=w1014, lo=w1131) -> ((hi.lo)=w1127:u16)
        n1023 = Join Numbers(hi=w1162, lo=w1163) -> ((hi.lo)=w1164:u32)
        n1024 = Join Numbers(hi=w1120, lo=w1120) -> ((hi.lo)=w1125:u16)
        n1025 = Join Numbers(hi=w1013, lo=w1120) -> ((hi.lo)=w1124:u16)
        n1026 = Join Numbers(hi=w1161, lo=w1160) -> ((hi.lo)=w1159:u32)
        n1027 = Join Numbers(hi=w1119, lo=w1119) -> ((hi.lo)=w1114:u16)
        n1028 = Join Numbers(hi=w1012, lo=w1119) -> ((hi.lo)=w1115:u16)
        n1029 = Join Numbers(hi=w1150, lo=w1151) -> ((hi.lo)=w1152:u32)
        n1030 = Join Numbers(hi=w1108, lo=w1108) -> ((hi.lo)=w1113:u16)
        n1031 = Join Numbers(hi=w1011, lo=w1108) -> ((hi.lo)=w1112:u16)
        n1032 = Join Numbers(hi=w1107, lo=w1107) -> ((hi.lo)=w1102:u16)
        n1033 = Join Numbers(hi=w1010, lo=w1107) -> ((hi.lo)=w1103:u16)
        n1034 = Join Numbers(hi=w1149, lo=w1148) -> ((hi.lo)=w1147:u32)
        n1035 = Join Numbers(hi=w1071, lo=w1071) -> ((hi.lo)=w1066:u16)
        n1036 = Join Numbers(hi=w1004, lo=w1071) -> ((hi.lo)=w1067:u16)
        n1037 = Join Numbers(hi=w1096, lo=w1096) -> ((hi.lo)=w1101:u16)
        n1038 = Join Numbers(hi=w1009, lo=w1096) -> ((hi.lo)=w1100:u16)
        n1039 = Join Numbers(hi=w1138, lo=w1139) -> ((hi.lo)=w1140:u32)
        n1040 = Join Numbers(hi=w1060, lo=w1060) -> ((hi.lo)=w1065:u16)
        n1041 = Join Numbers(hi=w1003, lo=w1060) -> ((hi.lo)=w1064:u16)
        n1042 = Join Numbers(hi=w1095, lo=w1095) -> ((hi.lo)=w1090:u16)
        n1043 = Join Numbers(hi=w1008, lo=w1095) -> ((hi.lo)=w1091:u16)
        n1044 = Join Numbers(hi=w1059, lo=w1059) -> ((hi.lo)=w1054:u16)
        n1045 = Join Numbers(hi=w1002, lo=w1059) -> ((hi.lo)=w1055:u16)
        n1046 = Join Numbers(hi=w1137, lo=w1136) -> ((hi.lo)=w1135:u32)
        n1047 = Join Numbers(hi=w1072, lo=w1072) -> ((hi.lo)=w1077:u16)
        n1048 = Join Numbers(hi=w1005, lo=w1072) -> ((hi.lo)=w1076:u16)
        n1049 = Join Numbers(hi=w1084, lo=w1084) -> ((hi.lo)=w1089:u16)
        n1050 = Join Numbers(hi=w1007, lo=w1084) -> ((hi.lo)=w1088:u16)
        n1051 = Join Numbers(hi=w1126, lo=w1127) -> ((hi.lo)=w1128:u32)
        n1052 = Join Numbers(hi=w1048, lo=w1048) -> ((hi.lo)=w1053:u16)
        n1053 = Join Numbers(hi=w1001, lo=w1048) -> ((hi.lo)=w1052:u16)
        n1054 = Join Numbers(hi=w1047, lo=w1047) -> ((hi.lo)=w1042:u16)
        n1055 = Join Numbers(hi=w1000, lo=w1047) -> ((hi.lo)=w1043:u16)
        n1056 = Join Numbers(hi=w1083, lo=w1083) -> ((hi.lo)=w1078:u16)
        n1057 = Join Numbers(hi=w1006, lo=w1083) -> ((hi.lo)=w1079:u16)
        n1058 = Join Numbers(hi=w1125, lo=w1124) -> ((hi.lo)=w1123:u32)
        n1059 = Bundle "Bundle"(w1172, w1172) -> (w1171:cluster{u32, u32})  [unwired: 1 in]
        n1060 = Join Numbers(hi=w1114, lo=w1115) -> ((hi.lo)=w1116:u32)
        n1061 = Join Numbers(hi=w1113, lo=w1112) -> ((hi.lo)=w1111:u32)
        n1062 = Join Numbers(hi=w1102, lo=w1103) -> ((hi.lo)=w1104:u32)
        n1063 = Bundle "Bundle"(w1164, w1164) -> (w1165:cluster{u32, u32})  [unwired: 1 in]
        n1064 = Join Numbers(hi=w1066, lo=w1067) -> ((hi.lo)=w1068:u32)
        n1065 = Join Numbers(hi=w1101, lo=w1100) -> ((hi.lo)=w1099:u32)
        n1066 = Join Numbers(hi=w1065, lo=w1064) -> ((hi.lo)=w1063:u32)
        n1067 = Join Numbers(hi=w1090, lo=w1091) -> ((hi.lo)=w1092:u32)
        n1068 = Join Numbers(hi=w1054, lo=w1055) -> ((hi.lo)=w1056:u32)
        n1069 = Bundle "Bundle"(w1159, w1159) -> (w1158:cluster{u32, u32})  [unwired: 1 in]
        n1070 = Join Numbers(hi=w1077, lo=w1076) -> ((hi.lo)=w1075:u32)
        n1071 = Bundle "Bundle"(w1152, w1152) -> (w1153:cluster{u32, u32})  [unwired: 1 in]
        n1072 = Join Numbers(hi=w1089, lo=w1088) -> ((hi.lo)=w1087:u32)
        n1073 = Join Numbers(hi=w1053, lo=w1052) -> ((hi.lo)=w1051:u32)
        n1074 = Join Numbers(hi=w1042, lo=w1043) -> ((hi.lo)=w1044:u32)
        n1075 = Join Numbers(hi=w1078, lo=w1079) -> ((hi.lo)=w1080:u32)
        n1076 = Bundle "Bundle"(w1147, w1147) -> (w1146:cluster{u32, u32})  [unwired: 1 in]
        n1077 = Bundle "Bundle"(w1140, w1140) -> (w1141:cluster{u32, u32})  [unwired: 1 in]
        n1078 = Bundle "Bundle"(w1135, w1135) -> (w1134:cluster{u32, u32})  [unwired: 1 in]
        n1079 = Bundle "Bundle"(w1128, w1128) -> (w1129:cluster{u32, u32})  [unwired: 1 in]
        n1080 = Bundle "Bundle"(w1123, w1123) -> (w1122:cluster{u32, u32})  [unwired: 1 in]
        n1081 = Bundle "Bundle"(w1116, w1116) -> (w1117:cluster{u32, u32})  [unwired: 1 in]
        n1082 = Bundle "Bundle"(w1111, w1111) -> (w1110:cluster{u32, u32})  [unwired: 1 in]
        n1083 = Bundle "Bundle"(w1104, w1104) -> (w1105:cluster{u32, u32})  [unwired: 1 in]
        n1084 = Bundle "Bundle"(w1068, w1068) -> (w1069:cluster{u32, u32})  [unwired: 1 in]
        n1085 = Bundle "Bundle"(w1099, w1099) -> (w1098:cluster{u32, u32})  [unwired: 1 in]
        n1086 = Bundle "Bundle"(w1063, w1063) -> (w1062:cluster{u32, u32})  [unwired: 1 in]
        n1087 = Bundle "Bundle"(w1092, w1092) -> (w1093:cluster{u32, u32})  [unwired: 1 in]
        n1088 = Bundle "Bundle"(w1056, w1056) -> (w1057:cluster{u32, u32})  [unwired: 1 in]
        n1089 = Bundle "Bundle"(w1075, w1075) -> (w1074:cluster{u32, u32})  [unwired: 1 in]
        n1090 = Bundle "Bundle"(w1087, w1087) -> (w1086:cluster{u32, u32})  [unwired: 1 in]
        n1091 = Bundle "Bundle"(w1051, w1051) -> (w1050:cluster{u32, u32})  [unwired: 1 in]
        n1092 = Bundle "Bundle"(w1044, w1044) -> (w1045:cluster{u32, u32})  [unwired: 1 in]
        n1093 = Bundle "Bundle"(w1080, w1080) -> (w1081:cluster{u32, u32})  [unwired: 1 in]
        n1094 = Build Array "Build Array"(cluster{u32, u32} {0, 0} ("element"), w1171) -> (w1021:cluster{u32, u32}[])
        n1095 = Build Array "Build Array"(cluster{u32, u32} {0, 0} ("element"), w1165) -> (w1022:cluster{u32, u32}[])
        n1096 = Build Array "Build Array"(cluster{u32, u32} {0, 0} ("element"), w1158) -> (w1023:cluster{u32, u32}[])
        n1097 = Build Array "Build Array"(cluster{u32, u32} {0, 0} ("element"), w1153) -> (w1024:cluster{u32, u32}[])
        n1098 = Build Array "Build Array"(cluster{u32, u32} {0, 0} ("element"), w1146) -> (w1025:cluster{u32, u32}[])
        n1099 = Build Array "Build Array"(cluster{u32, u32} {0, 0} ("element"), w1141) -> (w1026:cluster{u32, u32}[])
        n1100 = Build Array "Build Array"(cluster{u32, u32} {0, 0} ("element"), w1134) -> (w1027:cluster{u32, u32}[])
        n1101 = Build Array "Build Array"(cluster{u32, u32} {0, 0} ("element"), w1129) -> (w1028:cluster{u32, u32}[])
        n1102 = Build Array "Build Array"(cluster{u32, u32} {0, 0} ("element"), w1122) -> (w1029:cluster{u32, u32}[])
        n1103 = Build Array "Build Array"(cluster{u32, u32} {0, 0} ("element"), w1117) -> (w1030:cluster{u32, u32}[])
        n1104 = Build Array "Build Array"(cluster{u32, u32} {0, 0} ("element"), w1110) -> (w1031:cluster{u32, u32}[])
        n1105 = Build Array "Build Array"(cluster{u32, u32} {0, 0} ("element"), w1105) -> (w1032:cluster{u32, u32}[])
        n1106 = Build Array "Build Array"(cluster{u32, u32} {0, 0} ("element"), w1069) -> (w1038:cluster{u32, u32}[])
        n1107 = Build Array "Build Array"(cluster{u32, u32} {0, 0} ("element"), w1098) -> (w1033:cluster{u32, u32}[])
        n1108 = Build Array "Build Array"(cluster{u32, u32} {0, 0} ("element"), w1062) -> (w999:cluster{u32, u32}[])
        n1109 = Build Array "Build Array"(cluster{u32, u32} {0, 0} ("element"), w1093) -> (w1034:cluster{u32, u32}[])
        n1110 = Build Array "Build Array"(cluster{u32, u32} {0, 0} ("element"), w1057) -> (w1039:cluster{u32, u32}[])
        n1111 = Build Array "Build Array"(cluster{u32, u32} {0, 0} ("element"), w1074) -> (w1037:cluster{u32, u32}[])
        n1112 = Build Array "Build Array"(cluster{u32, u32} {0, 0} ("element"), w1086) -> (w1035:cluster{u32, u32}[])
        n1113 = Build Array "Build Array"(cluster{u32, u32} {0, 0} ("element"), w1050) -> (w1040:cluster{u32, u32}[])
        n1114 = Build Array "Build Array"(cluster{u32, u32} {0, 0} ("element"), w1045) -> (w1041:cluster{u32, u32}[])
        n1115 = Build Array "Build Array"(cluster{u32, u32} {0, 0} ("element"), w1081) -> (w1036:cluster{u32, u32}[])
        n1116 = property on="GL2" class="Bool (strict)"("Colors [4]"=w1026) -> ()  [unwired: 2 in, 2 out]
        n1117 = property on="MBL1" class="Bool (strict)"("Colors [4]"=w1021) -> ()  [unwired: 2 in, 2 out]
        n1118 = property on="DAL2" class="Bool (strict)"("Colors [4]"=w1022) -> ()  [unwired: 2 in, 2 out]
        n1119 = property on="LL" class="Bool (strict)"("Colors [4]"=w1023) -> ()  [unwired: 2 in, 2 out]
        n1120 = property on="B2L1" class="Bool (strict)"("Colors [4]"=w1024) -> ()  [unwired: 2 in, 2 out]
        n1121 = property on="B2L2" class="Bool (strict)"("Colors [4]"=w1025) -> ()  [unwired: 2 in, 2 out]
        n1122 = property on="GL1" class="Bool (strict)"("Colors [4]"=w1027) -> ()  [unwired: 2 in, 2 out]
        n1123 = property on="B3L2" class="Bool (strict)"("Colors [4]"=w1028) -> ()  [unwired: 2 in, 2 out]
        n1124 = property on="B3L1" class="Bool (strict)"("Colors [4]"=w1029) -> ()  [unwired: 2 in, 2 out]
        n1125 = property on="B2WICL" class="Bool (strict)"("Colors [4]"=w1030) -> ()  [unwired: 2 in, 2 out]
        n1126 = property on="MBL" class="Bool (strict)"("Colors [4]"=w1031) -> ()  [unwired: 2 in, 2 out]
        n1127 = property on="TBL" class="Bool (strict)"("Colors [4]"=w1032) -> ()  [unwired: 2 in, 2 out]
        n1128 = property on="SLL2" class="Bool (strict)"("Colors [4]"=w1033) -> ()  [unwired: 2 in, 2 out]
        n1129 = property on="SLL1" class="Bool (strict)"("Colors [4]"=w1034) -> ()  [unwired: 2 in, 2 out]
        n1130 = property on="KL2" class="Bool (strict)"("Colors [4]"=w1035) -> ()  [unwired: 2 in, 2 out]
        n1131 = property on="KL1" class="Bool (strict)"("Colors [4]"=w1036) -> ()  [unwired: 2 in, 2 out]
        n1132 = property on="PL" class="Bool (strict)"("Colors [4]"=w1037) -> ()  [unwired: 2 in, 2 out]
        n1133 = property on="LAL2" class="Bool (strict)"("Colors [4]"=w1038) -> ()  [unwired: 2 in, 2 out]
        n1134 = property on="LAL1" class="Bool (strict)"("Colors [4]"=w999) -> ()  [unwired: 2 in, 2 out]
        n1135 = property on="MBWICL" class="Bool (strict)"("Colors [4]"=w1039) -> ()  [unwired: 2 in, 2 out]
        n1136 = property on="MBL2" class="Bool (strict)"("Colors [4]"=w1040) -> ()  [unwired: 2 in, 2 out]
        n1137 = property on="DAL1" class="Bool (strict)"("Colors [4]"=w1041) -> ()  [unwired: 2 in, 2 out]
      }
    }
    n1138 = local read "Temperature"() -> (w814:u8)
    n1139 = In Range and Coerce(upper limit=30, x=w814, lower limit=10 ("y")) -> (In Range?=w813:bool)  [unwired: 1 out]
    n1140 = case shown="True" w813 {
      frame False {
      }
      frame True {
        w871 = i8 0 ("hi")
        w872 = i8 0 ("hi")
        w883 = i8 0 ("hi")
        w884 = i8 0 ("hi")
        w895 = i8 0 ("hi")
        w896 = i8 0 ("hi")
        w907 = i8 0 ("hi")
        w944 = i8 0 ("hi")
        w943 = i8 0 ("hi")
        w932 = i8 0 ("hi")
        w931 = i8 0 ("hi")
        w920 = i8 0 ("hi")
        w919 = i8 0 ("hi")
        w908 = i8 0 ("hi")
        w955 = i8 0 ("hi")
        w956 = i8 0 ("hi")
        w967 = i8 0 ("hi")
        w968 = i8 0 ("hi")
        w979 = i8 0 ("hi")
        w980 = i8 0 ("hi")
        w991 = i8 0 ("hi")
        w992 = i8 0 ("hi")
        n1141 = local read "Brightness\nDining Area Light 2"() -> (w865:u8)
        n1142 = local read "Brightness\nBedroom 2 \nLight 2"() -> (w862:u8)
        n1143 = local read "Brightness\nBedroom 2 \nW.I.C. Light"() -> (w857:u8)
        n1144 = local read "Brightness\nMaster Bedroom \nLight 1"() -> (w994:u8)
        n1145 = local read "Brightness\nGarage Light 2"() -> (w861:u8)
        n1146 = local read "Brightness\nBedroom 3 \nLight 2"() -> (w859:u8)
        n1147 = local read "Brightness\nBedroom 2 \nLight 1"() -> (w863:u8)
        n1148 = local read "Brightness\nMaster Bath \nLight"() -> (w856:u8)
        n1149 = local read "Brightness\nT&B Light"() -> (w855:u8)
        n1150 = local read "Brightness\nService Laundry \nLight 2"() -> (w854:u8)
        n1151 = local read "Brightness\nService Laundry \nLight 1"() -> (w853:u8)
        n1152 = local read "Brightness\nKitchen \nLight 2"() -> (w852:u8)
        n1153 = local read "Brightness\nBedroom 3 \nLight 1"() -> (w858:u8)
        n1154 = local read "Brightness\nGarage Light 1"() -> (w860:u8)
        n1155 = local read "Brightness\nLiving Area Light 1"() -> (w848:u8)
        n1156 = local read "Brightness\nLanai Light"() -> (w864:u8)
        n1157 = local read "Brightness\nLiving Area Light 2"() -> (w849:u8)
        n1158 = local read "Brightness\nKitchen \nLight 1"() -> (w851:u8)
        n1159 = local read "Brightness\n Porch Light"() -> (w850:u8)
        n1160 = local read "Brightness\nMaster Bedroom \nW.I.C. Light"() -> (w847:u8)
        n1161 = local read "Brightness\nMaster Bedroom \nLight 2"() -> (w846:u8)
        n1162 = local read "Brightness\nDining Area Light 1"() -> (w845:u8)
        n1163 = Join Numbers(hi=w991, lo=w865) -> ((hi.lo)=w988:u16)
        n1164 = Join Numbers(hi=w865, lo=w991) -> ((hi.lo)=w987:u16)
        n1165 = Join Numbers(hi=w980, lo=w864) -> ((hi.lo)=w983:u16)
        n1166 = Join Numbers(hi=w864, lo=w980) -> ((hi.lo)=w984:u16)
        n1167 = Join Numbers(hi=w992, lo=w994) -> ((hi.lo)=w996:u16)
        n1168 = Join Numbers(hi=w994, lo=w992) -> ((hi.lo)=w997:u16)
        n1169 = Join Numbers(hi=w979, lo=w863) -> ((hi.lo)=w976:u16)
        n1170 = Join Numbers(hi=w863, lo=w979) -> ((hi.lo)=w975:u16)
        n1171 = Join Numbers(hi=w968, lo=w862) -> ((hi.lo)=w971:u16)
        n1172 = Join Numbers(hi=w862, lo=w968) -> ((hi.lo)=w972:u16)
        n1173 = Join Numbers(hi=w988, lo=w987) -> ((hi.lo)=w986:u32)
        n1174 = Join Numbers(hi=w967, lo=w861) -> ((hi.lo)=w964:u16)
        n1175 = Join Numbers(hi=w861, lo=w967) -> ((hi.lo)=w963:u16)
        n1176 = Join Numbers(hi=w983, lo=w984) -> ((hi.lo)=w985:u32)
        n1177 = Join Numbers(hi=w996, lo=w997) -> ((hi.lo)=w998:u32)
        n1178 = Join Numbers(hi=w956, lo=w860) -> ((hi.lo)=w959:u16)
        n1179 = Join Numbers(hi=w860, lo=w956) -> ((hi.lo)=w960:u16)
        n1180 = Join Numbers(hi=w907, lo=w858) -> ((hi.lo)=w904:u16)
        n1181 = Join Numbers(hi=w858, lo=w907) -> ((hi.lo)=w903:u16)
        n1182 = Join Numbers(hi=w955, lo=w859) -> ((hi.lo)=w952:u16)
        n1183 = Join Numbers(hi=w859, lo=w955) -> ((hi.lo)=w951:u16)
        n1184 = Join Numbers(hi=w896, lo=w857) -> ((hi.lo)=w899:u16)
        n1185 = Join Numbers(hi=w857, lo=w896) -> ((hi.lo)=w900:u16)
        n1186 = Join Numbers(hi=w976, lo=w975) -> ((hi.lo)=w974:u32)
        n1187 = Join Numbers(hi=w971, lo=w972) -> ((hi.lo)=w973:u32)
        n1188 = Join Numbers(hi=w895, lo=w856) -> ((hi.lo)=w892:u16)
        n1189 = Join Numbers(hi=w856, lo=w895) -> ((hi.lo)=w891:u16)
        n1190 = Join Numbers(hi=w964, lo=w963) -> ((hi.lo)=w962:u32)
        n1191 = Join Numbers(hi=w884, lo=w855) -> ((hi.lo)=w887:u16)
        n1192 = Join Numbers(hi=w855, lo=w884) -> ((hi.lo)=w888:u16)
        n1193 = Join Numbers(hi=w908, lo=w851) -> ((hi.lo)=w911:u16)
        n1194 = Join Numbers(hi=w851, lo=w908) -> ((hi.lo)=w912:u16)
        n1195 = Join Numbers(hi=w883, lo=w854) -> ((hi.lo)=w880:u16)
        n1196 = Join Numbers(hi=w854, lo=w883) -> ((hi.lo)=w879:u16)
        n1197 = Join Numbers(hi=w959, lo=w960) -> ((hi.lo)=w961:u32)
        n1198 = Join Numbers(hi=w919, lo=w850) -> ((hi.lo)=w916:u16)
        n1199 = Join Numbers(hi=w850, lo=w919) -> ((hi.lo)=w915:u16)
        n1200 = Join Numbers(hi=w932, lo=w847) -> ((hi.lo)=w935:u16)
        n1201 = Join Numbers(hi=w847, lo=w932) -> ((hi.lo)=w936:u16)
        n1202 = Join Numbers(hi=w920, lo=w849) -> ((hi.lo)=w923:u16)
        n1203 = Join Numbers(hi=w849, lo=w920) -> ((hi.lo)=w924:u16)
        n1204 = Join Numbers(hi=w904, lo=w903) -> ((hi.lo)=w902:u32)
        n1205 = Join Numbers(hi=w872, lo=w853) -> ((hi.lo)=w875:u16)
        n1206 = Join Numbers(hi=w853, lo=w872) -> ((hi.lo)=w876:u16)
        n1207 = Bundle(w986, w986) -> (w989:cluster{u32, u32})  [unwired: 1 in]
        n1208 = Join Numbers(hi=w943, lo=w846) -> ((hi.lo)=w940:u16)
        n1209 = Join Numbers(hi=w846, lo=w943) -> ((hi.lo)=w939:u16)
        n1210 = Join Numbers(hi=w952, lo=w951) -> ((hi.lo)=w950:u32)
        n1211 = Join Numbers(hi=w899, lo=w900) -> ((hi.lo)=w901:u32)
        n1212 = Join Numbers(hi=w931, lo=w848) -> ((hi.lo)=w928:u16)
        n1213 = Join Numbers(hi=w848, lo=w931) -> ((hi.lo)=w927:u16)
        n1214 = Bundle(w985, w985) -> (w982:cluster{u32, u32})  [unwired: 1 in]
        n1215 = Bundle(w998, w998) -> (w995:cluster{u32, u32})  [unwired: 1 in]
        n1216 = Join Numbers(hi=w871, lo=w852) -> ((hi.lo)=w868:u16)
        n1217 = Join Numbers(hi=w852, lo=w871) -> ((hi.lo)=w867:u16)
        n1218 = Join Numbers(hi=w944, lo=w845) -> ((hi.lo)=w947:u16)
        n1219 = Join Numbers(hi=w845, lo=w944) -> ((hi.lo)=w948:u16)
        n1220 = Join Numbers(hi=w892, lo=w891) -> ((hi.lo)=w890:u32)
        n1221 = Join Numbers(hi=w887, lo=w888) -> ((hi.lo)=w889:u32)
        n1222 = Bundle(w974, w974) -> (w977:cluster{u32, u32})  [unwired: 1 in]
        n1223 = Join Numbers(hi=w911, lo=w912) -> ((hi.lo)=w913:u32)
        n1224 = Join Numbers(hi=w880, lo=w879) -> ((hi.lo)=w878:u32)
        n1225 = Join Numbers(hi=w916, lo=w915) -> ((hi.lo)=w914:u32)
        n1226 = Join Numbers(hi=w935, lo=w936) -> ((hi.lo)=w937:u32)
        n1227 = Bundle(w973, w973) -> (w970:cluster{u32, u32})  [unwired: 1 in]
        n1228 = Join Numbers(hi=w923, lo=w924) -> ((hi.lo)=w925:u32)
        n1229 = Join Numbers(hi=w875, lo=w876) -> ((hi.lo)=w877:u32)
        n1230 = Bundle(w962, w962) -> (w965:cluster{u32, u32})  [unwired: 1 in]
        n1231 = Join Numbers(hi=w940, lo=w939) -> ((hi.lo)=w938:u32)
        n1232 = Join Numbers(hi=w928, lo=w927) -> ((hi.lo)=w926:u32)
        n1233 = Bundle(w961, w961) -> (w958:cluster{u32, u32})  [unwired: 1 in]
        n1234 = Join Numbers(hi=w868, lo=w867) -> ((hi.lo)=w866:u32)
        n1235 = Join Numbers(hi=w947, lo=w948) -> ((hi.lo)=w949:u32)
        n1236 = Bundle(w902, w902) -> (w905:cluster{u32, u32})  [unwired: 1 in]
        n1237 = Bundle(w950, w950) -> (w953:cluster{u32, u32})  [unwired: 1 in]
        n1238 = Bundle(w901, w901) -> (w898:cluster{u32, u32})  [unwired: 1 in]
        n1239 = Bundle(w890, w890) -> (w893:cluster{u32, u32})  [unwired: 1 in]
        n1240 = Bundle(w889, w889) -> (w886:cluster{u32, u32})  [unwired: 1 in]
        n1241 = Build Array "Build Array"(cluster{u32, u32} {0, 0} ("element"), w989) -> (w824:cluster{u32, u32}[])
        n1242 = Bundle(w913, w913) -> (w910:cluster{u32, u32})  [unwired: 1 in]
        n1243 = Build Array "Build Array"(cluster{u32, u32} {0, 0} ("element"), w982) -> (w823:cluster{u32, u32}[])
        n1244 = Bundle(w878, w878) -> (w881:cluster{u32, u32})  [unwired: 1 in]
        n1245 = Build Array "Build Array"(cluster{u32, u32} {0, 0} ("element"), w995) -> (w825:cluster{u32, u32}[])
        n1246 = Bundle(w914, w914) -> (w917:cluster{u32, u32})  [unwired: 1 in]
        n1247 = Bundle(w937, w937) -> (w934:cluster{u32, u32})  [unwired: 1 in]
        n1248 = Bundle(w925, w925) -> (w922:cluster{u32, u32})  [unwired: 1 in]
        n1249 = Bundle(w877, w877) -> (w874:cluster{u32, u32})  [unwired: 1 in]
        n1250 = Bundle(w938, w938) -> (w941:cluster{u32, u32})  [unwired: 1 in]
        n1251 = Bundle(w926, w926) -> (w929:cluster{u32, u32})  [unwired: 1 in]
        n1252 = Build Array "Build Array"(cluster{u32, u32} {0, 0} ("element"), w977) -> (w826:cluster{u32, u32}[])
        n1253 = Bundle(w866, w866) -> (w869:cluster{u32, u32})  [unwired: 1 in]
        n1254 = Bundle(w949, w949) -> (w946:cluster{u32, u32})  [unwired: 1 in]
        n1255 = Build Array "Build Array"(cluster{u32, u32} {0, 0} ("element"), w970) -> (w828:cluster{u32, u32}[])
        n1256 = Build Array "Build Array"(cluster{u32, u32} {0, 0} ("element"), w965) -> (w827:cluster{u32, u32}[])
        n1257 = Build Array "Build Array"(cluster{u32, u32} {0, 0} ("element"), w958) -> (w830:cluster{u32, u32}[])
        n1258 = Build Array "Build Array"(cluster{u32, u32} {0, 0} ("element"), w905) -> (w831:cluster{u32, u32}[])
        n1259 = Build Array "Build Array"(cluster{u32, u32} {0, 0} ("element"), w953) -> (w829:cluster{u32, u32}[])
        n1260 = Build Array "Build Array"(cluster{u32, u32} {0, 0} ("element"), w898) -> (w832:cluster{u32, u32}[])
        n1261 = Build Array "Build Array"(cluster{u32, u32} {0, 0} ("element"), w893) -> (w835:cluster{u32, u32}[])
        n1262 = Build Array "Build Array"(cluster{u32, u32} {0, 0} ("element"), w886) -> (w834:cluster{u32, u32}[])
        n1263 = Build Array "Build Array"(cluster{u32, u32} {0, 0} ("element"), w910) -> (w838:cluster{u32, u32}[])
        n1264 = Build Array "Build Array"(cluster{u32, u32} {0, 0} ("element"), w881) -> (w833:cluster{u32, u32}[])
        n1265 = Build Array "Build Array"(cluster{u32, u32} {0, 0} ("element"), w917) -> (w839:cluster{u32, u32}[])
        n1266 = Build Array "Build Array"(cluster{u32, u32} {0, 0} ("element"), w934) -> (w842:cluster{u32, u32}[])
        n1267 = Build Array "Build Array"(cluster{u32, u32} {0, 0} ("element"), w922) -> (w840:cluster{u32, u32}[])
        n1268 = Build Array "Build Array"(cluster{u32, u32} {0, 0} ("element"), w874) -> (w837:cluster{u32, u32}[])
        n1269 = Build Array "Build Array"(cluster{u32, u32} {0, 0} ("element"), w941) -> (w843:cluster{u32, u32}[])
        n1270 = Build Array "Build Array"(cluster{u32, u32} {0, 0} ("element"), w929) -> (w841:cluster{u32, u32}[])
        n1271 = Build Array "Build Array"(cluster{u32, u32} {0, 0} ("element"), w869) -> (w836:cluster{u32, u32}[])
        n1272 = Build Array "Build Array"(cluster{u32, u32} {0, 0} ("element"), w946) -> (w844:cluster{u32, u32}[])
        n1273 = property on="MBWICL" class="Bool (strict)"("Colors [4]"=w842) -> ()  [unwired: 2 in, 2 out]
        n1274 = property on="DAL1" class="Bool (strict)"("Colors [4]"=w844) -> ()  [unwired: 2 in, 2 out]
        n1275 = property on="MBL2" class="Bool (strict)"("Colors [4]"=w843) -> ()  [unwired: 2 in, 2 out]
        n1276 = property on="PL" class="Bool (strict)"("Colors [4]"=w839) -> ()  [unwired: 2 in, 2 out]
        n1277 = property on="MBL1" class="Bool (strict)"("Colors [4]"=w825) -> ()  [unwired: 2 in, 2 out]
        n1278 = property on="DAL2" class="Bool (strict)"("Colors [4]"=w824) -> ()  [unwired: 2 in, 2 out]
        n1279 = property on="LL" class="Bool (strict)"("Colors [4]"=w823) -> ()  [unwired: 2 in, 2 out]
        n1280 = property on="LAL2" class="Bool (strict)"("Colors [4]"=w840) -> ()  [unwired: 2 in, 2 out]
        n1281 = property on="B2L1" class="Bool (strict)"("Colors [4]"=w826) -> ()  [unwired: 2 in, 2 out]
        n1282 = property on="KL1" class="Bool (strict)"("Colors [4]"=w838) -> ()  [unwired: 2 in, 2 out]
        n1283 = property on="LAL1" class="Bool (strict)"("Colors [4]"=w841) -> ()  [unwired: 2 in, 2 out]
        n1284 = property on="B2L2" class="Bool (strict)"("Colors [4]"=w828) -> ()  [unwired: 2 in, 2 out]
        n1285 = property on="GL2" class="Bool (strict)"("Colors [4]"=w827) -> ()  [unwired: 2 in, 2 out]
        n1286 = property on="TBL" class="Bool (strict)"("Colors [4]"=w834) -> ()  [unwired: 2 in, 2 out]
        n1287 = property on="SLL2" class="Bool (strict)"("Colors [4]"=w833) -> ()  [unwired: 2 in, 2 out]
        n1288 = property on="SLL1" class="Bool (strict)"("Colors [4]"=w837) -> ()  [unwired: 2 in, 2 out]
        n1289 = property on="KL2" class="Bool (strict)"("Colors [4]"=w836) -> ()  [unwired: 2 in, 2 out]
        n1290 = property on="GL1" class="Bool (strict)"("Colors [4]"=w830) -> ()  [unwired: 2 in, 2 out]
        n1291 = property on="B3L2" class="Bool (strict)"("Colors [4]"=w829) -> ()  [unwired: 2 in, 2 out]
        n1292 = property on="MBL" class="Bool (strict)"("Colors [4]"=w835) -> ()  [unwired: 2 in, 2 out]
        n1293 = property on="B2WICL" class="Bool (strict)"("Colors [4]"=w832) -> ()  [unwired: 2 in, 2 out]
        n1294 = property on="B3L1" class="Bool (strict)"("Colors [4]"=w831) -> ()  [unwired: 2 in, 2 out]
      }
    }
  }
  "Open Door" <- FALSE ("Open Door")
  "Fire Alarm" <- FALSE ("ABC")
